vi "Main.vi"(11 "Module Admin":refnum<class "Delacor_lib_QMH_Module Admin.lvclass">) -> ()   [LabVIEW 2023, in "Panther Dashboard.lvlib"]
doc: "Panther Dashboard For DQMH®\n\nDeveloped and maintained by:\nPantherLAB\n\nMain Contributor- Developer:\n\n» Enrique Noé Arias\n\nBrainstorming & Code Reviews:\n\n» Matthias Baudot\n» Fabiola De La Cueva\n» Christopher Farmer\n» Cyril Gambini\n» Joerg Hampel\n» Olivier Jourdan\n» Cesar Muñoz\n» Darren Nattinger\n» Luis Orozco\n» Sam Taggart\n» Diego Torres\n\n<b>Note:</b> This VI was modified by the <b>Validate DQMH Module</b> tool to add a call to the Error Reported VI at the end of the 'Exit' MHL frame."
uses:
  Panther Dashboard.lvlib
  <vilib>/Delacor/Delacor QMH/Libraries/Module Admin_class/Delacor_lib_QMH_Module Admin.lvclass
  Module Data--cluster.ctl
  Maps List and refs--cluster.ctl
  <vilib>/National Instruments/Tree Map/Tree Map Data.ctl
  DQMH Modules Info--cluster.ctl
  Module type--enum.ctl
  Project References--cluster.ctl
  Selection Type--enum.ctl
  References Updated Argument--cluster.ctl
  Launch DQMH Scripting Tools Argument--cluster.ctl
  DQMH Tools Menu--enum.ctl
  <vilib>/Delacor/Delacor QMH/Libraries/Message Queue_class/Delacor_lib_QMH_Message Queue.lvclass/Delacor_lib_QMH_Message Queue.ctl
  Execute Default Event Request Argument--cluster.ctl
  Tree DQMH Selection Argument--cluster.ctl
  Expand Results Argument--cluster.ctl
  Scan DQMH Modules Argument--cluster.ctl
  Stop Argument--cluster.ctl
  Generate Project Documentation Argument--cluster.ctl
  Set App Theme Argument--cluster.ctl
  Show About Argument--cluster.ctl
  Update Module ID Argument--cluster.ctl
  Save Library Description Argument--cluster.ctl
  Save VI Description Argument--cluster.ctl
  Open Documentation Argument--cluster.ctl
  Save Project Documentation Argument--cluster.ctl
  Save Module Spec Argument--cluster.ctl
  Public VIs names--enum.ctl
  <vilib>/Delacor/Delacor QMH/Libraries/Module Admin_class/Delacor_lib_QMH_Module Admin.lvclass/Delacor_lib_QMH_Module Admin.ctl
  <vilib>/Delacor/Delacor QMH/Libraries/Message Queue_class/Delacor_lib_QMH_Enqueue Message (Single).vi
  <vilib>/Delacor/Delacor QMH/Libraries/Module Admin_class/Delacor_lib_QMH_Get External Launch.vi
  Panther Dashboard--global.vi
  <vilib>/Platform/browser.llb/Open URL in Default Browser (path).vi
  <vilib>/Utility/error.llb/Error Cluster From Error Code.vi
  <vilib>/ErrorRing/Error Ring.xnode
  <vilib>/Delacor/Delacor QMH/Libraries/Message Queue_class/Delacor_lib_QMH_Message Queue.lvclass
  <vilib>/National Instruments/Tree Map/Tree Map.lvlib
  <vilib>/Delacor/Delacor QMH/Libraries/Scripting API/DQMH_Scripting API.lvlib
  ContextHelp/ContextHelp.lvlib
panel:
  out "error out":errorcluster
  in  "Context Help Panther":bool caption="Doc Editor"
  in  "Add Event":bool
  in  "Remove Event":bool caption="Remove"
  in  "Convert Event":bool caption="Convert"
  in  "Rename Event":bool caption="Rename"
  in  "Add Helper Loop to Module":bool
  in  "Add New Module":bool caption="Add"
  in  "Rename Module":bool caption="Rename"
  in  "Validate Module":bool caption="Validate"
  in  "Create Module Template":bool caption="Template"
  in  "Add Unit Test Module":bool caption="Unit Test"
  in  "Create RT Tester Module":bool caption="RT Tester"
  in  "Open Antidoc Output":bool caption="Open"
  in  "Generate Antidoc":bool caption="Antidoc"
  in  "About Panther":bool caption="About"
  in  "Theme Panther":bool caption="Theme"
  in  "Projects":string(combo)
  in  "Targets":string(combo)
  in  "Save Module Spec":bool
  in  "Scan All":bool
  in  "Search":bool caption="Scan Project"
  in  "Include Dependencies":bool
  in  "Expand Results":bool
  in  "Module ID":i32=-1 min=-1 max=1000 step=1 format="Module ID %d"
  in  "Modules Tree":string(tree)
  out "antidoc":bool
  out "Panther Indicator":bool
  out "Process Indicator":bool
  out "Event Indicator":bool
  out "Status":string
  out "Progress":u16(slide) scale=-1.0..1.0
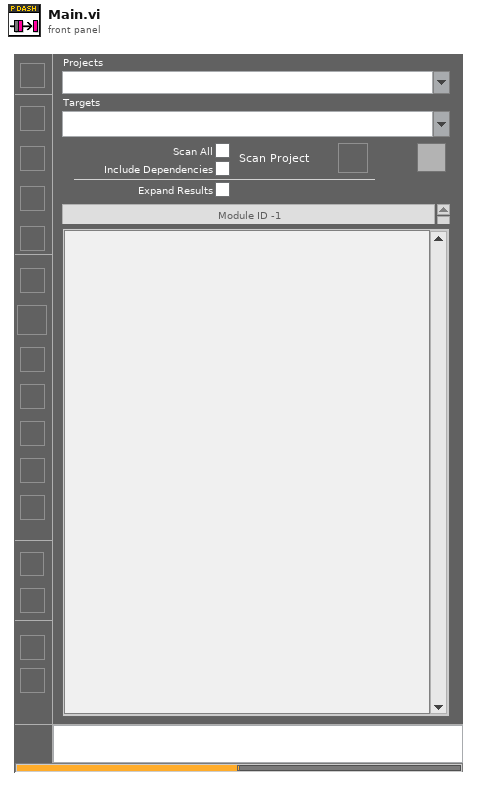
[diagram p1: front panel]
types:
  T1 = typedef "Panther Dashboard.lvlib/Broadcast Events--cluster.ctl" = cluster{"Module Did Init":refnum<user-event>, "Status Updated":refnum<user-event>, "Error Reported":refnum<user-event>, "Module Did Stop":refnum<user-event>, "Update Module Execution Status":refnum<user-event>, "References Updated":refnum<user-event>, "Projects Updated":refnum<user-event>, "Targets Updated":refnum<user-event>, "Progress updated":refnum<user-event>, "Scale Updated":refnum<user-event>, "Connector Pane Updated":refnum<user-event>, "Documentation Updated":refnum<user-event>, "Module Type Updated":refnum<user-event>, "Theme Updated":refnum<user-event>, "Project Description Updated":refnum<user-event>}
  T2 = typedef "Panther Dashboard.lvlib/Request Events--cluster.ctl" = cluster{"Stop Module":refnum<user-event>, "Show Panel":refnum<user-event>, "Hide Panel":refnum<user-event>, "Get Module Execution Status":refnum<user-event>, "Show Diagram":refnum<user-event>, "Scan DQMH Modules":refnum<user-event>, "Tree DQMH Selection":refnum<user-event>, "Open Module API Tester":refnum<user-event>, "Execute Default Event Request":refnum<user-event>, "Expand Results":refnum<user-event>, "Launch DQMH Scripting Tools":refnum<user-event>, "Generate Project Documentation":refnum<user-event>, "Set App Theme":refnum<user-event>, "Show About":refnum<user-event>, "Update Module ID":refnum<user-event>, "Save Library Description":refnum<user-event>, "Save VI Description":refnum<user-event>, "Open Documentation":refnum<user-event>, "Save Project Documentation":refnum<user-event>, "Register controls Mouse Enter":refnum<user-event>, "Save Module Spec":refnum<user-event>}
  T3 = typedef "ContextHelp.lvlib/Broadcast Events--cluster.ctl" = cluster{"Module Did Init":refnum<user-event>, "Status Updated":refnum<user-event>, "Error Reported":refnum<user-event>, "Module Did Stop":refnum<user-event>, "Update Module Execution Status":refnum<user-event>}
  T4 = typedef "Panther Dashboard.lvlib/Selection Type--enum.ctl" = enum16{"Module", "Public API", "Broadcast", "Request", "Request and Wait for Reply"}
  T5 = typedef "Panther Dashboard.lvlib/Module Data--cluster.ctl" = cluster{"Maps":T6, "DQMH Scan Results":T8, "Current Selection":cluster{"VI Ref":refnum<vi>, "DQMH Lib Ref":refnum<vi>}, "Module type":T9, "Module ID":i32, "Theme":bool, "Broadcast?":bool}
  T6 = typedef "Panther Dashboard.lvlib/Maps List and refs--cluster.ctl" = cluster{"Tree Map":T7, "References Map":map{string, refnum<vi>}}
  T7 = typedef "Tree Map.lvlib/Tree Map Data.ctl" = map{string, cluster{"Child Paths Set":set{string}, "Name":string, "Data":string, "Attributes":map{string, string}}}
  T8 = typedef "Panther Dashboard.lvlib/DQMH Modules Info--cluster.ctl" = cluster{"All DQMH Modules Refs":refnum<vi>[], "All Modules Descriptions":string[], "All Modules type":T9[], "Project References":T10, "Dependencies":bool[]}
  T9 = typedef "Panther Dashboard.lvlib/Module type--enum.ctl" = enum16{"Singleton", "Cloneable"}
  T10 = typedef "Panther Dashboard.lvlib/Project References--cluster.ctl" = cluster{"Project Ref":refnum<vi>, "Project Name":string, "Target":refnum<vi>, "App Ref":refnum<vi>}
  T11 = typedef "Panther Dashboard.lvlib/References Updated Argument--cluster.ctl" = cluster{"Modules":refnum<vi>[], "Modules Types":T9[], "Application Instance":refnum<vi>, "Dependencies":bool[]}
  T12 = enum8{"Enabled", "Disabled", "Disabled and Grayed Out"}
  T13 = typedef "Panther Dashboard.lvlib/Launch DQMH Scripting Tools Argument--cluster.ctl" = cluster{"Scripting Tool":T14}
  T14 = typedef "Panther Dashboard.lvlib/DQMH Tools Menu--enum.ctl" = enum16{"Create New DQMH Event", "Remove DQMH Event", "Convert DQMH Event", "Rename DQMH Event", "Add New DQMH Module", "Create RT Tester", "Rename DQMH Module", "Validate DQMH Module", "Create DQMH Module Template", "New DQMH  Unit Test", "Add Helper Loop to DQMH Module"}
  T15 = typedef "Panther Dashboard.lvlib/Execute Default Event Request Argument--cluster.ctl" = cluster{"Event Name":string}
  T16 = typedef "Panther Dashboard.lvlib/Tree DQMH Selection Argument--cluster.ctl" = cluster{"Tree DQMH Sel":string}
  T17 = typedef "Panther Dashboard.lvlib/Expand Results Argument--cluster.ctl" = cluster{"Expand?":bool}
  T18 = typedef "Panther Dashboard.lvlib/Scan DQMH Modules Argument--cluster.ctl" = cluster{"Include Dependencies":bool, "Scan All":bool, "Project":string, "Target":string}
  T19 = enum32{"invalid lock state", "Not Locked", "Locked (No Password)", "Password-protected"}
  T20 = typedef "Panther Dashboard.lvlib/Stop Argument--cluster.ctl" = cluster{"Origin":string, "Exit via Stop Module Req?":bool, "Wait for Module to stop?":bool}
  T21 = typedef "Panther Dashboard.lvlib/Generate Project Documentation Argument--cluster.ctl" = cluster{"Boolean":bool}
  T22 = typedef "Panther Dashboard.lvlib/Set App Theme Argument--cluster.ctl" = cluster{"Theme":bool}
  T23 = typedef "Panther Dashboard.lvlib/Show About Argument--cluster.ctl" = cluster{"Boolean":bool}
  T24 = typedef "Panther Dashboard.lvlib/Update Module ID Argument--cluster.ctl" = cluster{"New ID":i32}
  T25 = typedef "Panther Dashboard.lvlib/Save Library Description Argument--cluster.ctl" = cluster{"Library Description":string}
  T26 = typedef "Panther Dashboard.lvlib/Save VI Description Argument--cluster.ctl" = cluster{"VI Description":string}
  T27 = typedef "Panther Dashboard.lvlib/Open Documentation Argument--cluster.ctl" = cluster{"Boolean":bool}
  T28 = typedef "Panther Dashboard.lvlib/Save Project Documentation Argument--cluster.ctl" = cluster{"Project Description":string}
  T29 = typedef "Panther Dashboard.lvlib/Save Module Spec Argument--cluster.ctl" = cluster{"Boolean":bool}
  T30 = typedef "Panther Dashboard.lvlib/Public VIs names--enum.ctl" = enum16{"Start Module.vi", "Synchronize Module Events.vi", "Obtain Broadcast Events for Registration.vi", "Null Broadcast Events--constant.vi", "Stop Module.vi"}
  T31 = enum32{"Invalid", "Standard", "Closed", "Hidden", "Minimized", "Maximized"}
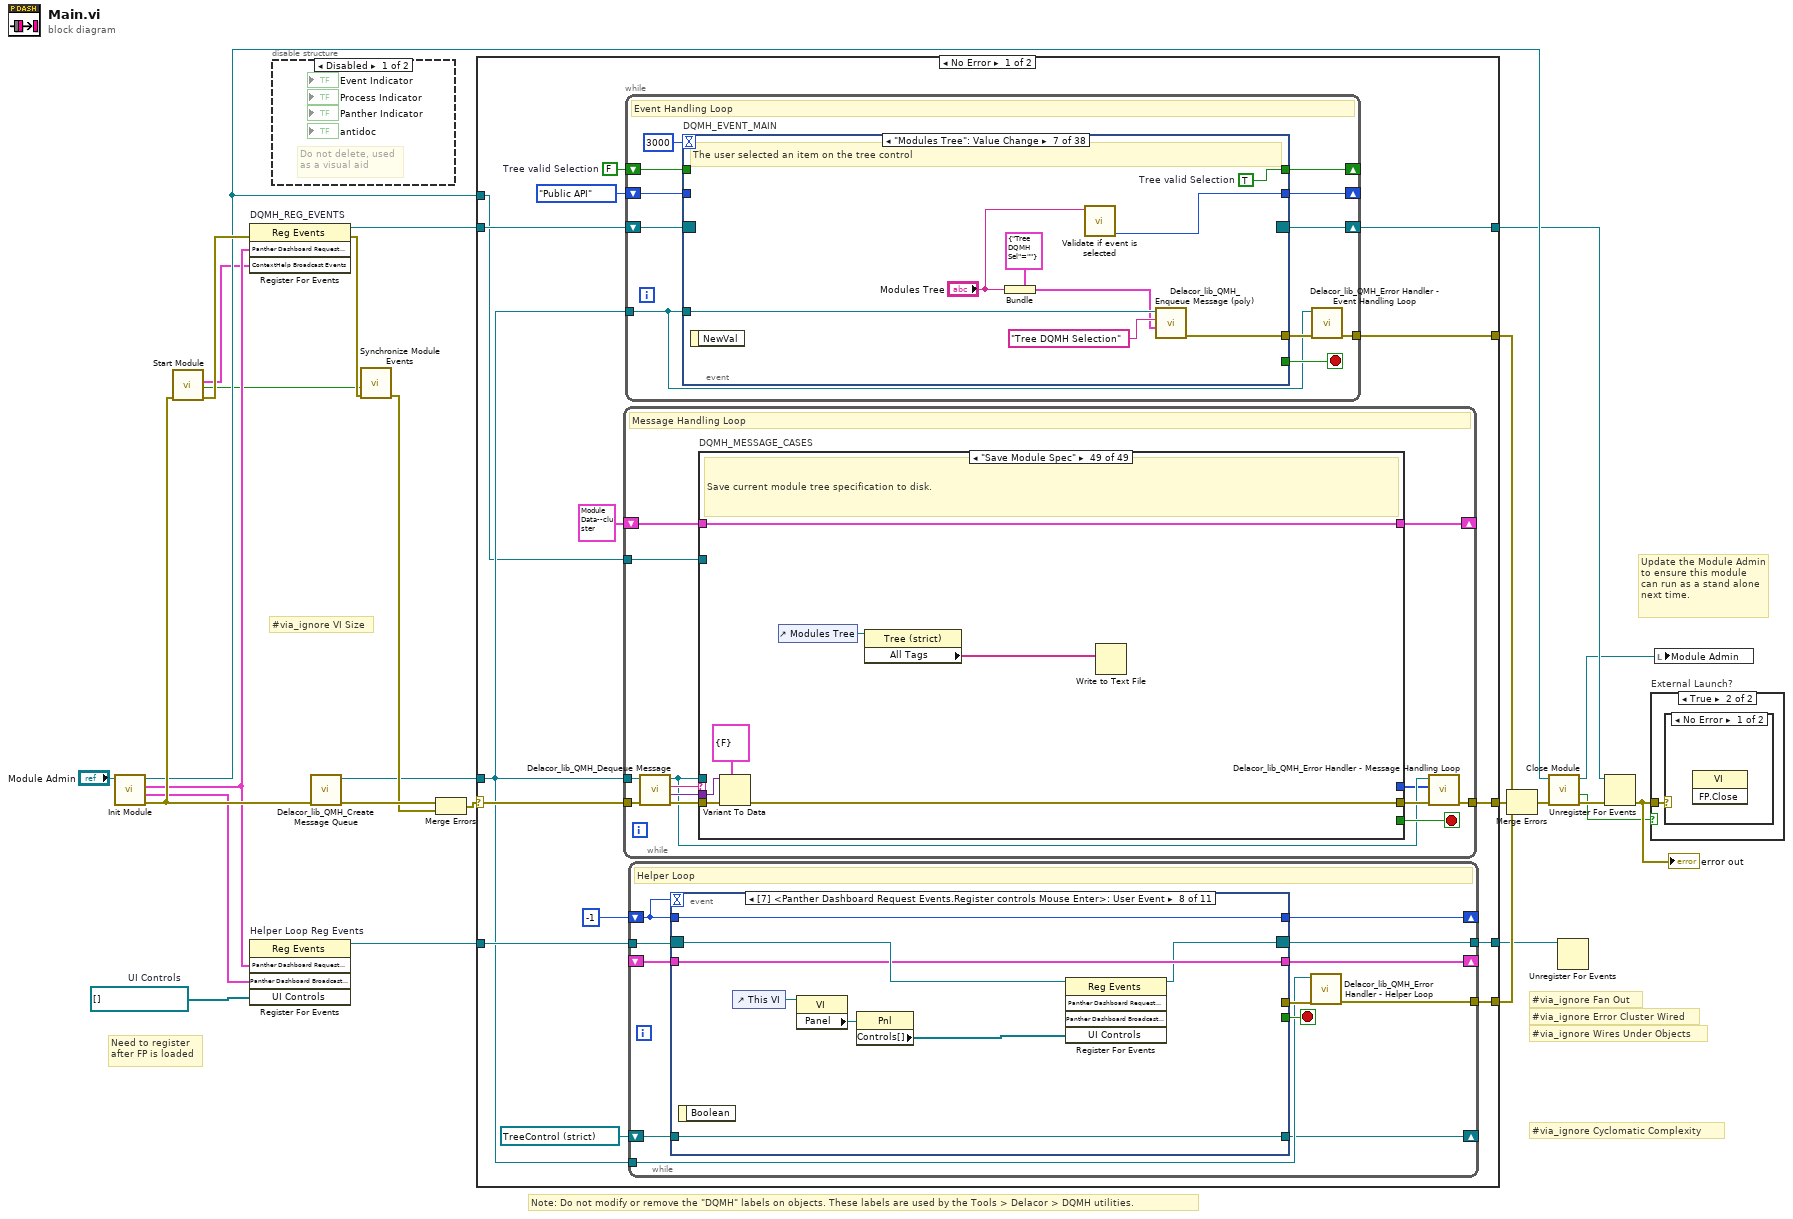
[diagram p0: block diagram]
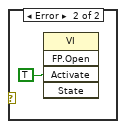
[diagram p4: hidden frame]
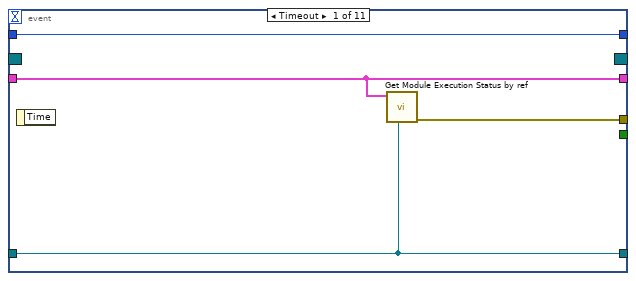
[diagram p5: hidden frame]
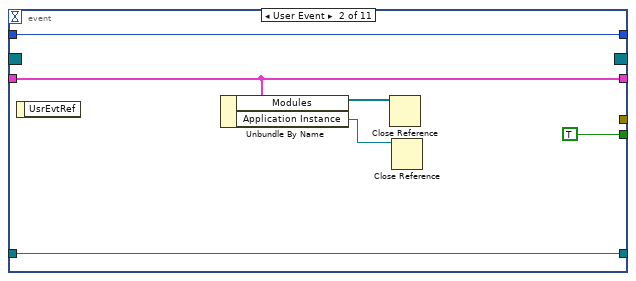
[diagram p6: hidden frame]
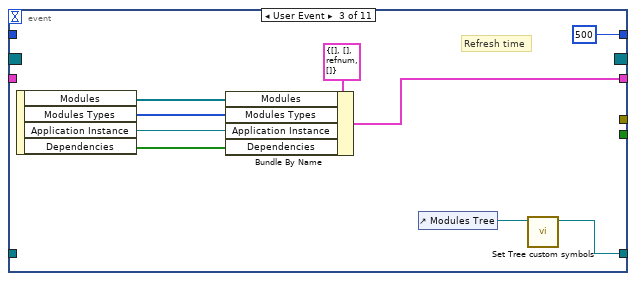
[diagram p7: hidden frame]
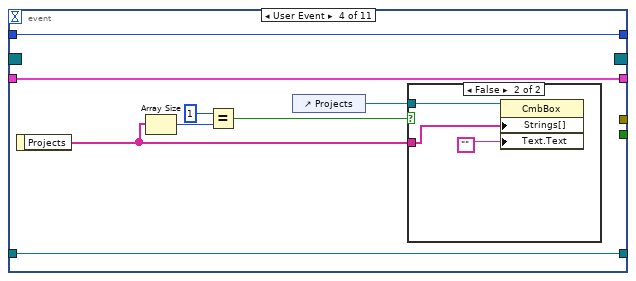
[diagram p8: hidden frame]
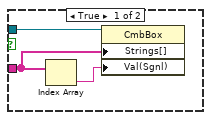
[diagram p9: hidden frame]
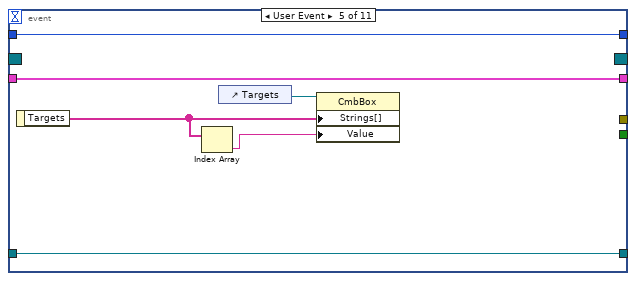
[diagram p10: hidden frame]
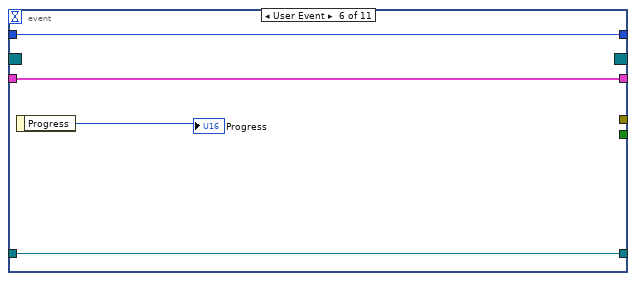
[diagram p11: hidden frame]
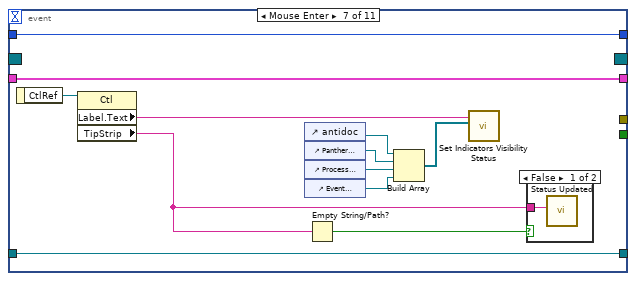
[diagram p12: hidden frame]
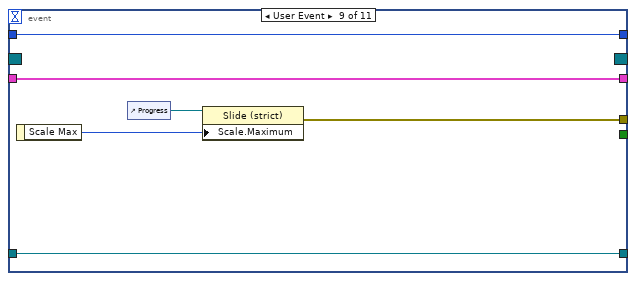
[diagram p14: hidden frame]
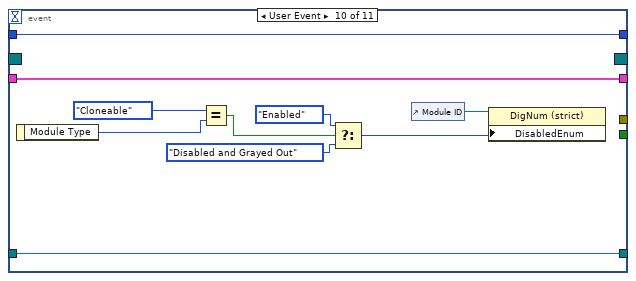
[diagram p15: hidden frame]
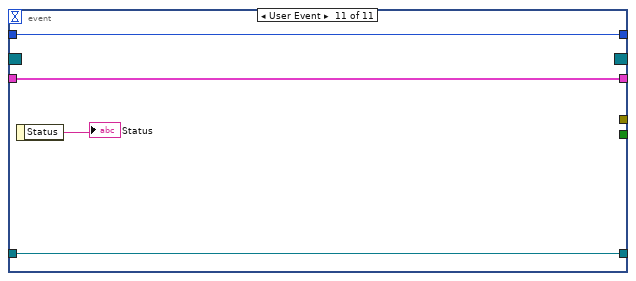
[diagram p16: hidden frame]
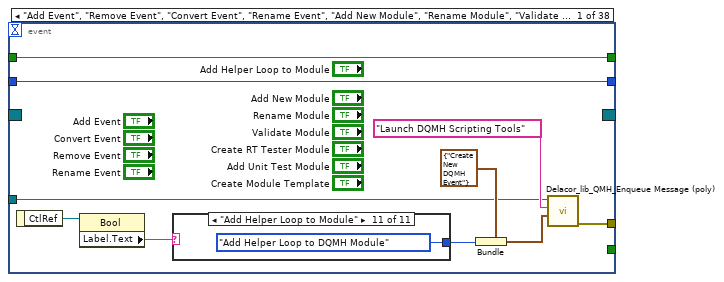
[diagram p17: hidden frame]
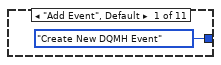
[diagram p18: hidden frame]
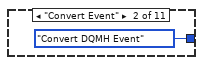
[diagram p19: hidden frame]
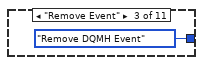
[diagram p20: hidden frame]
diagram:
  w1 = refnum<vi>[] []  # UI Controls
  # "Need to register\nafter FP is loaded"
  # "#via_ignore VI Size"
  # "#via_ignore Fan Out"
  # "#via_ignore Cyclomatic Complexity"
  # "#via_ignore Wires Under Objects"
  # "#via_ignore Error Cluster Wired"
  # "Note: Do not modify or remove the \"DQMH\" labels on objects. These labels are used by the Tools > Delacor > DQMH utilities."
  # "Update the Module Admin to ensure this module can run as a stand alone next time."
  n1 = call "Init Module.vi"("Singleton Module Admin in"="Module Admin") -> ("error out"=w15:errorcluster, "Panther Dashboard Broadcast Events"=w4:T1, "Panther Dashboard Request Events"=w5:T2, "Singleton Module Admin out"=w14:refnum<class "Delacor_lib_QMH_Module Admin.lvclass">)  [unwired: 7 in]
  n2 = call "Start Module.vi"("error in"=w15) -> ("error out"=w17:errorcluster, "Wait for Event Sync?"=w3:bool, "ContextHelp Broadcast Events"=w2:T3)  [unwired: 7 in, 1 out]
  n3 = register-events "DQMH_REG_EVENTS"(error in=w17, w5, w2) -> (reference out=w12:refnum<event-registration>, error out=w18:errorcluster)  [unwired: 1 in]
  n4 = register-events "Helper Loop Reg Events"(w5, w4, w1) -> (reference out=w7:refnum<event-registration>)  [unwired: 2 in, 1 out]
  n5 = disable-structure shown="Disabled" {
    frame Disabled {
      # "Do not delete, used\nas a visual aid"
    }
    frame Enabled {
    }
  }
  n6 = call <vilib>:"Delacor_lib_QMH_Create Message Queue.vi"("error in"=w15) -> ("error out"=w21:errorcluster, "Message Queue"=w11:refnum<class "Delacor_lib_QMH_Message Queue.lvclass">)  [unwired: 9 in]
  n7 = call "Synchronize Module Events.vi"("error in"=w18, "Wait for Event Sync?"=w3) -> ("error out"=w16:errorcluster)  [unwired: 9 in]
  n8 = Merge Errors(w21, w16) -> (w20:errorcluster)
  n9 = case shown="No Error" w20 {
    selector: w20 -> [w39 w924]
    tunnel: [w41 w923] -> w26
    tunnel: [w37 w922] -> w13
    tunnel: w12 -> [w35 w922]
    tunnel: w11 -> [w31 w918]
    tunnel: [w40 _] -> w24
    tunnel: w14 -> [w28 w919]
    tunnel: w7 -> [w34 w917]
    tunnel: [w33 w917] -> w6
    tunnel: [w38 _] -> w19
    frame No Error {
      w30 = FALSE  # Tree valid Selection
      n10 = while {
        tunnel: w31 -> [w466]
        shift-right: [w470] -> _
        shift-left: T5 {"Maps"={"Tree Map"={}, "References Map"={}}, "DQMH Scan Results"={"All DQMH Modules Refs"=[], "All Modules Descriptions"=[], "All Modules type"=[], "Project References"={"Project Ref"=refnum, "Project Name"="", "Target"=refnum, "App Ref"=refnum}, "Dependencies"=[]}, "Current Selection"={"VI Ref"=refnum, "DQMH Lib Ref"=refnum}, "Module type"=enum."Singleton", "Module ID"=0, "Theme"=FALSE, "Broadcast?"=FALSE} ("Data Cluster") -> [w471]
        tunnel: w39 -> [w474]
        tunnel: [w472] -> w41
        tunnel: w28 -> [w464]
        stop <- w469 stop-if-true
        # "Message Handling Loop"
        n11 = call-dynamic "Delacor_lib_QMH_Dequeue Message.vi"("error in"=w474, "Message Queue in"=w466) -> ("error out"=w473:errorcluster, "Message Data"=w467:variant, "Message"=w468:string, "Message Queue out"=w465:refnum<class "Delacor_lib_QMH_Message Queue.lvclass">)  [unwired: 6 in]
        n12 = case "DQMH_MESSAGE_CASES" shown="\"Save Module Spec\"" w468 {
          selector: w468 -> [_ _ _ _ w525 _ _ _ _ _ _ _ _ _ _ _ _ _ _ _ _ _ _ _ _ _ _ _ _ _ _ _ _ _ _ _ _ _ _ _ _ _ _ _ _ _ _ w896 _]
          tunnel: w465 -> [_ _ _ _ _ _ _ _ _ _ _ _ _ _ _ _ _ _ _ _ _ _ _ _ _ _ _ _ _ _ _ _ _ _ _ _ _ _ _ _ _ _ _ _ _ w865 w888 _ _]
          tunnel: w473 -> [w496 w501 w510 w522 w530 w537 w544 w551 w560 w567 w573 w579 w586 w593 w598 w604 w606 w613 w615 w620 w634 w647 w669 w676 w682 w687 w693 w700 w707 w720 w722 w732 w741 w749 w764 w766 w771 w781 w798 w807 w817 w831 w849 w860 w862 w872 w894 w898 w915]
          tunnel: [w490 w501 w508 w521 w528 w536 w544 w551 w559 w566 w572 w578 w585 w592 w599 w603 w606 w613 w615 w621 w632 w646 w670 w677 w681 w686 w692 w699 w706 w718 w722 w730 w737 w748 w763 w766 w770 w780 w798 w805 w815 w829 w848 w858 w862 w868 w891 w899 w914] -> w475
          tunnel: w471 -> [w476 w500 w505 w520 w527 w534 w543 w550 w558 w565 w571 w577 w584 w591 w597 w602 w605 w612 w614 w619 w627 w644 w668 w674 w680 w685 w691 w698 w705 w709 w721 w729 w736 w747 w759 w765 w769 w778 w797 w801 w810 w823 w838 w854 w861 w867 w880 w897 w911]
          tunnel: [w487 w500 w504 w519 w527 w534 w543 w550 w558 w565 w571 w577 w584 w591 w597 w602 w605 w612 w614 w619 w627 w644 w668 w674 w680 w685 w691 w696 w705 w709 w721 w724 w736 w743 w755 w765 w769 w778 w797 w801 w808 w822 w838 w854 w861 w867 w880 w897 w911] -> w470
          tunnel: [_ _ _ _ _ _ _ _ _ _ _ _ _ _ _ _ _ _ _ _ _ _ _ _ _ _ _ _ _ _ _ _ _ _ _ _ _ _ _ _ _ _ _ _ _ _ w887 _ _] -> w469
          tunnel: w467 -> [_ _ w507 _ w526 _ _ _ _ _ _ _ _ _ _ _ _ _ _ _ w630 _ _ _ _ _ _ w697 w704 w717 _ w728 w735 w746 w762 _ _ _ _ w803 w813 w827 w847 w857 _ w866 w886 _ w913]
          tunnel: w464 -> [w488 _ _ _ _ _ _ _ _ _ _ _ _ _ _ _ _ _ _ _ _ _ _ _ _ _ _ _ _ _ _ _ _ _ _ _ _ _ _ _ _ _ _ _ _ w864 w881 _ _]
          tunnel: [_ _ _ _ _ _ _ _ _ _ _ _ _ _ _ _ _ _ _ _ _ i32[] [5000, 1026, 43] ("specific error code to clear (0: all)") _ _ _ _ _ _ _ _ _ _ _ _ _ _ _ _ _ _ _ _ _ _ _ _ _ _ _] -> w463
          frame "Initialize" {
            w478 = "Panther Dashboard for DQMH" ("format string")
            # "Initialize - Any operation that needs to be done before the module can receive messages. Synchronize Caller Events.vi will inform Start Module.vi that the module has launched and is ready to receive messages. Module Did Init.vi will broadcast that the module initialized."
            n13 = call "Synchronize Caller Events.vi"("error in (no error)"=w496, "Singleton Module Admin in"=w488) -> ("error out"=w495:errorcluster)  [unwired: 8 in, 1 out]
            n14 = property on="Modules Tree" class="Tree (strict)"("Allow Item Drag"=TRUE ("Drag/Drop:Allow Dragging"), "SelColor"=u32 8355711) -> ()  [unwired: 2 in, 2 out]
            n15 = call "Module Name--constant.vi"() -> ("Module Name"=w485:string)  [unwired: 11 in]
            n16 = call "Module Did Init.vi"("error in (no error)"=w495, "Initialized?"=TRUE, "Origin"=w485) -> ("error out"=w494:errorcluster)  [unwired: 8 in]
            n17 = control-ref of="Projects"() -> (w481:refnum<vi>)
            n18 = call "Scan For App Projects.vi"("error in"=w494, "Init?"=TRUE, "Projects Ref"=w481) -> ("error out"=w493:errorcluster)  [unwired: 8 in]
            n19 = call "Read Theme from Config.vi"("error in"=w493) -> ("error out"=w492:errorcluster, "Theme"=w477:bool)  [unwired: 9 in]
            n20 = local write "Theme Panther"(w477) -> ()
            n21 = call "Set App Theme.vi"("error in"=w492, "Theme"=w477) -> ("error out"=w491:errorcluster)  [unwired: 9 in]
            n22 = control-ref of="This VI"() -> (w479:refnum<vi>)
            n23 = disable-structure shown="Disabled" {
              disable-tunnel: [w499 _] -> w489
              disable-tunnel: w479 -> [w498 _]
              disable-tunnel: w478 -> [w497 _]
              frame Disabled {
                n24 = call "Set Panel Initial State.vi"("Title"=w497, "Main Vi Ref"=w498) -> ("error out"=w499:errorcluster)  [unwired: 9 in]
              }
              frame Enabled {
              }
            }
            n25 = Bundle By Name(cluster=w476, "Module ID"=-1) -> (w487:T5)
            n26 = call "Status Updated.vi"("Status"=w478) -> ()  [unwired: 10 in, 1 out]
            n27 = Merge Errors(w489, w491) -> (w490:errorcluster)
          }
          frame "--------MODULE-----------" {
          }
          frame "Scan DQMH Modules" {
            # "Scan DQMH Modules in the project and fill 2 maps one with the Vi References and the another one with the list of DQMH modules on the project"
            n28 = Variant To Data(error in=w510, type=T18 {"Include Dependencies"=FALSE, "Scan All"=FALSE, "Project"="", "Target"=""} ("Scan DQMH Modules Argument"), Variant=w507) -> (data=w502:T18, error out=w509:errorcluster)
            n29 = call <vilib>:"Set Busy.vi"("error in (no error)"=w509) -> ()  [unwired: 9 in, 2 out]
            n30 = control-ref of="Modules Tree"() -> (w503:refnum<vi>)
            n31 = call "Scan DQMH Modules and create Maps.vi"("TreeControl in"=w503, "Data Cluster In"=w505, "error in"=w509, "Scan DQMH Modules Argument"=w502) -> ("error out"=w508:errorcluster, "Data Cluster Out"=w504:T5)  [unwired: 6 in]
            n32 = call <vilib>:"Unset Busy.vi"("error in (no error)"=w508) -> ()  [unwired: 10 in, 1 out]
          }
          frame "Refresh Module" {
            # "User right click a module and selected Refresh module"
            n33 = Unbundle By Name(w520) -> ("DQMH Scan Results.Project References.App Ref"=w513:refnum<vi>, "Current Selection.DQMH Lib Ref"=w514:refnum<vi>, "Maps.Tree Map"=w516:T7, "Maps.References Map"=w515:map{string, refnum<vi>})
            n34 = local read "Expand Results"() -> (w512:bool)
            n35 = control-ref of="Modules Tree"() -> (w511:refnum<vi>)
            n36 = call "Refresh Current DQMH Module.vi"("TreeControl in"=w511, "App Ref"=w513, "Expand Results"=w512, "DQMH Lib Ref"=w514, "error in"=w522, "References Map"=w515, "Tree Map In"=w516) -> ("error out"=w521:errorcluster, "map ref out"=w518:map{string, refnum<vi>}, "Tree Map out"=w517:T7)  [unwired: 2 in]
            n37 = Bundle By Name(cluster=w520, "Maps.Tree Map"=w517, "Maps.References Map"=w518) -> (w519:T5)
          }
          frame "Refresh Targets" {
            # "When the User selects a Project triggers this task to scan all the targets available"
            n38 = Variant To Data(error in=w530, type=w525, Variant=w526) -> (data=w524:string, error out=w529:errorcluster)
            n39 = call "Get all Targets.vi"("error in"=w529, "Project Selection"=w524) -> ("error out"=w528:errorcluster, "Targets"=w523:string[])  [unwired: 8 in]
            n40 = call "Targets Updated.vi"("Targets"=w523) -> ()  [unwired: 10 in, 1 out]
          }
          frame "Drag VI" {
            # "This is the functionality alowing drag and drop the current selection to your code, you can edit DQMH code using panther Dashboard as it was the Project Explorer"
            n41 = Unbundle By Name(w534) -> ("DQMH Scan Results.Project References.App Ref"=w533:refnum<vi>, "DQMH Scan Results.Project References.Target"=w532:refnum<vi>, "Current Selection.VI Ref"=w531:refnum<vi>)
            n42 = call "Drop Event into subVI.vi"("Current Selection.VI Ref"=w531, "Target"=w532, "App Ref"=w533) -> ("error out"=w535:errorcluster)  [unwired: 8 in]
            n43 = Merge Errors(w535, w537) -> (w536:errorcluster)
          }
          frame "Where is this module being Launched?" {
            # "Find all the VIS calling the Start Module.vi of the selected module library"
            n44 = Unbundle By Name(w543) -> ("Theme"=w542:bool, "DQMH Scan Results.Project References.App Ref"=w541:refnum<vi>, "DQMH Scan Results.Project References.Target"=w540:refnum<vi>, "Current Selection.DQMH Lib Ref"=w539:refnum<vi>)
            n45 = call "Find some Public API VI.vi"("Theme"=w542, "Framework VI to Find"=Public_VIs_names--enum."Start Module.vi", "Library in"=w539, "Target"=w540, "App Ref"=w541) -> ()  [unwired: 7 in]
          }
          frame "Where is this module being Stopped?" {
            # "Find all the VIS calling the Obtain broadcast events for registration of the selected module library"
            n46 = Unbundle By Name(w550) -> ("Theme"=w548:bool, "DQMH Scan Results.Project References.App Ref"=w547:refnum<vi>, "DQMH Scan Results.Project References.Target"=w546:refnum<vi>, "Current Selection.DQMH Lib Ref"=w545:refnum<vi>)
            n47 = call "Find some Public API VI.vi"("Theme"=w548, "Framework VI to Find"=Public_VIs_names--enum."Stop Module.vi", "Library in"=w545, "Target"=w546, "App Ref"=w547) -> ()  [unwired: 7 in]
          }
          frame "Open Module API Tester" {
            # "If nothing selected use the first DQMH module"
            # "Open the API Tester from the current DQMH Module Selected"
            n48 = Unbundle By Name(w558) -> ("DQMH Scan Results.Project References.App Ref"=w557:refnum<vi>, "DQMH Scan Results.All DQMH Modules Refs"=w556:refnum<vi>[], "Current Selection.DQMH Lib Ref"=w552:refnum<vi>)
            n49 = Index Array(array=w556) -> (element=w554:refnum<vi>)  [unwired: 1 in]
            n50 = Not A Number/Path/Refnum?(number/path/refnum=w552) -> (NaN/Path/Refnum?=w555:bool)
            n51 = Select(t=w554, s=w555, f=w552) -> (s? t:f=w553:refnum<vi>)
            n52 = call "Open API Tester.vi"("error in"=w560, "DQMH Library Ref"=w553, "Application Instance"=w557) -> ("error out"=w559:errorcluster)  [unwired: 8 in]
          }
          frame "Create Custom --error.vi" {
            n53 = Unbundle By Name(w565) -> ("Module type"=w561:T9, "Current Selection.DQMH Lib Ref"=w564:refnum<vi>, "Theme"=w563:bool, "DQMH Scan Results.Project References.App Ref"=w562:refnum<vi>)
            n54 = call "Error Code Dialog.vi"("Module type"=w561, "error in"=w567, "App Ref"=w562, "Theme"=w563, "Library in"=w564) -> ("error out"=w566:errorcluster)  [unwired: 6 in]
          }
          frame "Create Custom --constant.vi" {
            n55 = Unbundle By Name(w571) -> ("Current Selection.DQMH Lib Ref"=w570:refnum<vi>, "Theme"=w569:bool, "DQMH Scan Results.Project References.App Ref"=w568:refnum<vi>)
            n56 = call "Custom Constant Dialog.vi"("error in"=w573, "App Ref"=w568, "Theme"=w569, "Library in"=w570) -> ("error out"=w572:errorcluster)  [unwired: 7 in]
          }
          frame "Edit 'Module Name--constant.vi' value" {
            # "Sometimes we need to update or modify the 'Module Name--constant.vi' value and we need to go to this vi, open it's block diagram and change the constant value, close the vi and save it, this script does exactly that."
            n57 = Unbundle By Name(w577) -> ("Theme"=w574:bool, "DQMH Scan Results.Project References.App Ref"=w576:refnum<vi>, "Current Selection.DQMH Lib Ref"=w575:refnum<vi>)
            n58 = call "Script Edit Module Name.vi"("Theme"=w574, "error in"=w579, "Library in"=w575, "App Ref"=w576) -> ("error out"=w578:errorcluster)  [unwired: 7 in]
          }
          frame "Edit 'Module Timeout--constant.vi' value" {
            w580 = FALSE  # Restore to Default
            # "Sometimes we need to update or modify the 'Module Name--constant.vi' value and we need to go to this vi, open it's block diagram and change the constant value, close the vi and save it, this script does exactly that."
            n59 = Unbundle By Name(w584) -> ("Theme"=w581:bool, "DQMH Scan Results.Project References.App Ref"=w583:refnum<vi>, "Current Selection.DQMH Lib Ref"=w582:refnum<vi>)
            n60 = call "Script Module Timeout.vi"("Restore to Default"=w580, "Theme"=w581, "error in"=w586, "Library in"=w582, "App Ref"=w583) -> ("error out"=w585:errorcluster)  [unwired: 6 in]
          }
          frame "Restore Timeout to Default (5000ms)" {
            w587 = TRUE  # Restore to Default
            # "Restore Timeout to Default DQMH Framework value (5000ms)"
            n61 = Unbundle By Name(w591) -> ("Theme"=w588:bool, "DQMH Scan Results.Project References.App Ref"=w590:refnum<vi>, "Current Selection.DQMH Lib Ref"=w589:refnum<vi>)
            n62 = call "Script Module Timeout.vi"("Restore to Default"=w587, "Theme"=w588, "error in"=w593, "Library in"=w589, "App Ref"=w590) -> ("error out"=w592:errorcluster)  [unwired: 6 in]
          }
          frame "Find Module in project" {
            # "Find the selected module in project explorer"
            n63 = Unbundle By Name(w597) -> ("Current Selection.DQMH Lib Ref"=w596:refnum<vi>, "DQMH Scan Results.Project References.Project Ref"=w595:refnum<vi>, "DQMH Scan Results.All DQMH Modules Refs"=w594:refnum<vi>[])
            n64 = call "Find Library in Project.vi"("error in"=w598, "DQMH Modules Refs"=w594, "Project Ref"=w595, "DQMH Lib Ref"=w596) -> ("error out"=w599:errorcluster)  [unwired: 7 in]
          }
          frame "Open File Library on Disk" {
            # "Open current Module Library selection on the file system"
            n65 = Unbundle By Name(w602) -> ("Current Selection.DQMH Lib Ref"=w601:refnum<vi>)
            n66 = property class="Library"(reference=w601) -> ("Path"=w600:path)  [unwired: 1 in, 2 out]
            n67 = call "Open File on Disk.vi"("error in"=w604, "file or directory path"=w600) -> ("error out"=w603:errorcluster)  [unwired: 9 in]
          }
          frame "---------BROADCASTS---------" {
          }
          frame "Find Code registered to this module's broadcasts" {
            # "Find all the VIS calling the Obtain broadcast events for registration of the selected module library"
            n68 = Unbundle By Name(w612) -> ("Theme"=w610:bool, "DQMH Scan Results.Project References.App Ref"=w609:refnum<vi>, "DQMH Scan Results.Project References.Target"=w608:refnum<vi>, "Current Selection.DQMH Lib Ref"=w607:refnum<vi>)
            n69 = call "Find some Public API VI.vi"("Theme"=w610, "Framework VI to Find"=Public_VIs_names--enum."Obtain Broadcast Events for Registration.vi", "Library in"=w607, "Target"=w608, "App Ref"=w609) -> ()  [unwired: 7 in]
          }
          frame "---------REQUEST--------------" {
          }
          frame "Locate Event on Main" {
            # "Find the selected event vi on the owing DQMH Module, if it is a reques we highlight its frame, if it is a broadcast we highlight where the broadcast is being triggered"
            n70 = Unbundle By Name(w619) -> ("DQMH Scan Results.Project References.App Ref"=w617:refnum<vi>, "Current Selection.VI Ref"=w618:refnum<vi>, "Broadcast?"=w616:bool)
            n71 = call "Find Event Frame.vi"("error in"=w620, "Broadcast?"=w616, "VI in"=w618, "Application Instance"=w617) -> ("error out"=w621:errorcluster)  [unwired: 7 in]
          }
          frame "Execute Default Event Request" {
            # "Execute Default Event"
            n72 = Variant To Data(error in=w634, type=T15 {"Event Name"=""} ("Execute Default Event Request Argument"), Variant=w630) -> (data=w628:T15, error out=w633:errorcluster)
            n73 = Unbundle By Name(w627) -> ("DQMH Scan Results.Project References.App Ref"=w626:refnum<vi>, "Current Selection.DQMH Lib Ref"=w625:refnum<vi>, "Module ID"=w623:i32, "Module type"=w622:T9)
            n74 = Unbundle By Name(w628) -> ("Event Name"=w624:string)
            n75 = call "Execute Default event.vi"("Module type"=w622, "Module ID"=w623, "Event"=w624, "DQMH Library Ref"=w625, "application Instance"=w626) -> ("error out"=w631:errorcluster)  [unwired: 6 in]
            n76 = Merge Errors(w633, w631) -> (w632:errorcluster)
          }
          frame "Search for Event Callers / listeners" {
            # "1026-Invalid Ref\n43- Operation\n canceled by user\n5000- something\nrandom happening\non DQMH Scripting\nAPI"
            # "Search for this event callers"
            n77 = Unbundle By Name(w644) -> ("DQMH Scan Results.Project References.Project Ref"=w638:refnum<vi>, "Current Selection.VI Ref"=w643:refnum<vi>, "Theme"=w635:bool, "Broadcast?"=w636:bool)
            n78 = Select(t="Searching code registered to broadcast selection" ("Status"), s=w636, f="Searching for Event Callers" ("Status")) -> (s? t:f=w639:string)
            n79 = call "Status Updated.vi"("error in (no error)"=w647, "Status"=w639) -> ("error out"=w645:errorcluster)  [unwired: 9 in]
            n80 = case shown="True" w636 {
              tunnel: w645 -> [w652 w659]
              tunnel: [w651 w658] -> w646
              tunnel: w643 -> [w650 w655]
              tunnel: [w649 w657] -> w642
              tunnel: w638 -> [w648 w656]
              frame False {
                # "Requests"
                n81 = call <vilib>:"Get Callers of Request VI in Project.vi"("error in"=w652, "Request VI"=w650, "Project"=w648) -> ("error out"=w651:errorcluster, "Request VI Callers"=w649:refnum<vi>[])  [unwired: 7 in]
              }
              frame True {
                # "Broadcast"
                n82 = Two Button Dialog(message="This is an exhaustive task that can take up to minutes, do you wish to continue?") -> (T button?=w654:bool)  [unwired: 2 in]
                n83 = case shown="True" w654 {
                  tunnel: w659 -> [w660 w665]
                  tunnel: [w660 w664] -> w658
                  tunnel: [_ w663] -> w657
                  tunnel: w656 -> [_ w662]
                  tunnel: w655 -> [_ w661]
                  frame False {
                  }
                  frame True {
                    n84 = call <vilib>:"Get VIs Registered for Broadcast in Project.vi"("error in"=w665, "Broadcast VI"=w661, "Project"=w662) -> ("error out"=w664:errorcluster, "VIs Registered for Broadcast"=w663:refnum<vi>[])  [unwired: 7 in]
                  }
                }
              }
            }
            n85 = call <vilib>:"Set Busy.vi"("error in (no error)"=w645) -> ()  [unwired: 9 in, 2 out]
            n86 = call <vilib>:"Unset Busy.vi"("error in (no error)"=w646) -> ()  [unwired: 10 in, 1 out]
            n87 = call "Start Call to results window.vi"("Find Broadcast?"=w636, "Request VI Callers"=w642, "Event"=w643, "Theme"=w635) -> ()  [unwired: 8 in]
          }
          frame "Open VI on Disk" {
            # "Open current event selection on the file system"
            n88 = Unbundle By Name(w668) -> ("Current Selection.VI Ref"=w667:refnum<vi>)
            n89 = property class="VI"(reference=w667) -> ("Path"=w666:path)  [unwired: 1 in, 2 out]
            n90 = call "Open File on Disk.vi"("error in"=w669, "file or directory path"=w666) -> ("error out"=w670:errorcluster)  [unwired: 9 in]
          }
          frame "Open Event Arguments" {
            # "Open The event selected DQMH Arguments, also open the Event BD to do edits on it"
            n91 = Unbundle By Name(w674) -> ("Current Selection.VI Ref"=w673:refnum<vi>)
            n92 = property on="Property Node" class="VI"(reference=w673, error in=w676, "BDWin.Open"=TRUE ("Block Diagram Window:Open")) -> (reference out=w671:refnum<vi>, error out=w675:errorcluster)
            n93 = call "Open Event Arguments.vi"("error in"=w675, "VI Refnum"=w671) -> ("error out"=w677:errorcluster)  [unwired: 9 in]
          }
          frame "Set Custom Timeout" {
            n94 = Unbundle By Name(w680) -> ("Theme"=w678:bool, "Current Selection.VI Ref"=w679:refnum<vi>)
            n95 = call "Script Request and Wait For Reply Custom Timeout.vi"("error in"=w682, "VI Ref"=w679, "Theme"=w678) -> ("error out"=w681:errorcluster)  [unwired: 8 in]
          }
          frame "Restore to Module's Timeout" {
            # "The requests and wait for reply utilize a notifier created on the fly to get the module's answer (Reply), there is a Wait for Notifier funtion with a timeout input, by default all the DQMH modules has a constant vi with a 5000 ms timeout value, what this script does is to make sure that the selected request utilizes Module Timeout--constant.vi no matter what the value it is inside."
            n96 = Unbundle By Name(w685) -> ("Current Selection.DQMH Lib Ref"=w683:refnum<vi>, "Current Selection.VI Ref"=w684:refnum<vi>)
            n97 = call "Script Request and Wait For Reply Restore Timeout.vi"("error in"=w687, "VI Ref"=w684, "DQMH Lib Ref"=w683) -> ("error out"=w686:errorcluster)  [unwired: 8 in]
          }
          frame "Open Front Panel" {
            # "User Selection 'Open Front Panel'"
            n98 = Unbundle By Name(w691) -> ("Current Selection.VI Ref"=w690:refnum<vi>)
            n99 = invoke class="VI" method="FP.Open"(reference=w690, error in=w693, "Activate"=TRUE ("Activate?"), "State"=T31."Standard") -> (error out=w692:errorcluster)  [unwired: 1 in, 4 out]
          }
          frame "Module ID Update" {
            # "Module ID Control has value change"
            n100 = Variant To Data(error in=w700, type=0 ("Module ID"), Variant=w697) -> (data=w695:i32, error out=w699:errorcluster)
            n101 = Bundle By Name(cluster=w698, "Module ID"=w695) -> (w696:T5)
          }
          frame "Expand or Close" {
            # "Expand or Close DQMH Tree control"
            n102 = Variant To Data(error in=w707, type=T17 {"Expand?"=FALSE} ("Expand or Close Argument"), Variant=w704) -> (data=w702:T17, error out=w706:errorcluster)
            n103 = Unbundle By Name(w702) -> ("Expand?"=w701:bool)
            n104 = invoke on="Modules Tree" class="Tree (strict)" method="Open/Close.Open/Close All"("Open"=w701) -> ()  [unwired: 3 in, 4 out]
          }
          frame "Launch DQMH Scripting Tools" {
            # "Launch the DQMH Scripting Tools"
            n105 = Variant To Data(error in=w720, type=T13 {"Scripting Tool"=enum."Create New DQMH Event"} ("Launch DQMH Scripting Tools Argument"), Variant=w717) -> (data=w715:T13, error out=w719:errorcluster)
            n106 = Unbundle By Name(w715) -> ("Scripting Tool"=w710:T14)
            n107 = Unbundle By Name(w709) -> ("DQMH Scan Results.Project References.Project Name"=w713:string, "DQMH Scan Results.Project References.App Ref"=w714:refnum<vi>, "Current Selection.DQMH Lib Ref"=w708:refnum<vi>)
            n108 = Format Into String(format string="DQMH Tool: %s being executed ", w710) -> (resulting string=w712:string)  [unwired: 2 in, 1 out]
            n109 = call "Status Updated.vi"("Status"=w712) -> ()  [unwired: 10 in, 1 out]
            n110 = call "Launch DQMH Tools by menu.vi"("Project"=w713, "Application Instance"=w714, "error in"=w719, "Module Ref"=w708, "DQMH Tools"=w710) -> ("error out"=w718:errorcluster)  [unwired: 6 in]
          }
          frame "-------PANTHER---------" {
          }
          frame "Set App Theme" {
            # "Set Panther Dashboard Theme"
            n111 = Variant To Data(error in=w732, type=T22 {"Theme"=FALSE} ("Set App Theme Argument"), Variant=w728) -> (data=w726:T22, error out=w731:errorcluster)
            n112 = Unbundle By Name(w726) -> ("Theme"=w723:bool)
            n113 = control-ref of="This VI"() -> (w725:refnum<vi>)
            n114 = Bundle By Name(cluster=w729, "Theme"=w723) -> (w724:T5)
            n115 = call "Set Theme.vi"("Dark?"=w723, "VI in"=w725) -> ()  [unwired: 10 in]
            n116 = call "Theme Updated.vi"("Theme"=w723) -> ()  [unwired: 10 in, 1 out]
            n117 = call "Save Theme in config.vi"("error in"=w731, "Theme"=w723) -> ("error out"=w730:errorcluster)  [unwired: 9 in]
          }
          frame "Show About" {
            # "Show About project"
            n118 = Variant To Data(error in=w741, type=T23 {"Boolean"=FALSE} ("Show About Argument"), Variant=w735) -> (error out=w738:errorcluster)  [unwired: 1 out]
            n119 = control-ref of="This VI"() -> (w733:refnum<vi>)
            n120 = call "Hide VI Panel.vi"("error in (no error)"=w738, "VI"=w733) -> ("error out"=w740:errorcluster)  [unwired: 9 in]
            n121 = call "About Panther Dashboard.vi"("error in"=w740) -> ("error out"=w739:errorcluster)  [unwired: 10 in]
            n122 = call "Open VI Panel.vi"("error in (no error)"=w739, "VI"=w733) -> ("error out"=w737:errorcluster)  [unwired: 9 in]
          }
          frame "Update Module ID" {
            # "Update the Current Module ID"
            n123 = Variant To Data(error in=w749, type=T24 {"New ID"=-1} ("Update Module ID Argument"), Variant=w746) -> (data=w744:T24, error out=w748:errorcluster)
            n124 = Unbundle By Name(w744) -> ("New ID"=w742:i32)
            n125 = Bundle By Name(cluster=w747, "Module ID"=w742) -> (w743:T5)
          }
          frame "Tree DQMH Selection" {
            # "There is a new selection of the DQMH Tree list, need to search and update indicators acordanly."
            n126 = Unbundle By Name(w759) -> ("Maps.Tree Map"=w758:T7, "Maps.References Map"=w757:map{string, refnum<vi>}, "DQMH Scan Results"=w756:T8)
            n127 = Variant To Data(error in=w764, type=T16 {"Tree DQMH Sel"=""} ("Tree DQMH Selection Argument"), Variant=w762) -> (data=w760:T16, error out=w763:errorcluster)
            n128 = Unbundle By Name(w760) -> ("Tree DQMH Sel"=w753:string)
            n129 = call "Get List Information.vi"("List Selection"=w753, "DQMH Scan Info"=w756, "References Map"=w757, "Tree Map"=w758) -> ("Broadcast?"=w752:bool, "Vi out"=w751:refnum<vi>, "Module type"=w750:T9, "DQMH Lib"=w754:refnum<vi>)  [unwired: 4 in]
            n130 = Bundle By Name(cluster=w759, "Current Selection.DQMH Lib Ref"=w754, "Module type"=w750, "Current Selection.VI Ref"=w751, "Broadcast?"=w752) -> (w755:T5)
          }
          frame "-------PROJECT----------" {
          }
          frame "Open Project Folder" {
            n131 = Unbundle By Name(w769) -> ("DQMH Scan Results.Project References.Project Ref"=w768:refnum<vi>)
            n132 = property class="Project"(reference=w768) -> ("Path"=w767:path)  [unwired: 1 in, 2 out]
            n133 = call "Open File on Disk.vi"("error in"=w771, "file or directory path"=w767) -> ("error out"=w770:errorcluster)  [unwired: 9 in]
          }
          frame "Show Project DQMH Info" {
            n134 = Unbundle By Name(w778) -> ("DQMH Scan Results.All Modules type"=w772:T9[], "Theme"=w775:bool, "DQMH Scan Results.Project References.App Ref"=w777:refnum<vi>, "DQMH Scan Results.All DQMH Modules Refs"=w773:refnum<vi>[])
            n135 = call "Status Updated.vi"("Status"="Getting Project info") -> ("error out"=w779:errorcluster)  [unwired: 10 in]
            n136 = Empty Array?(array=w773) -> (empty?=w774:bool)
            n137 = case shown="False" w774 {
              tunnel: w773 -> [w787 _]
              tunnel: w781 -> [w792 w796]
              tunnel: w777 -> [w786 _]
              tunnel: [w790 w794] -> w780
              tunnel: w775 -> [w785 _]
              tunnel: w779 -> [_ _]
              tunnel: w772 -> [w782 _]
              frame False {
                # "Project has been scanned"
                n138 = call "Script Parse Project Modules Constants.vi"("App Ref"=w786, "error in"=w792, "All DQMH Modules Refs"=w787) -> ("error out"=w791:errorcluster, "Project info Results"=w783:string[][])  [unwired: 7 in]
                n139 = call "Hide Panel.vi"("error in (no error)"=w791) -> ("error out"=w789:errorcluster)  [unwired: 10 in]
                n140 = call "Insert Module Types.vi"("All Modules types"=w782, "Project info Results In"=w783) -> ("Project info Results Out"=w784:string[][])  [unwired: 9 in]
                n141 = call "Display Project Info Results.vi"("Theme"=w785, "error in"=w789, "Project Results"=w784) -> ("error out"=w788:errorcluster)  [unwired: 8 in]
                n142 = call "Show Panel.vi"("error in (no error)"=w788) -> ("error out"=w790:errorcluster)  [unwired: 10 in]
              }
              frame True {
                n143 = invoke on="Projects" class="CmbBox" method="ObjHighlight"(error in=w796) -> (error out=w795:errorcluster)  [unwired: 2 in, 2 out]
                n144 = invoke on="Search" class="Bool" method="ObjHighlight"(error in=w795) -> (error out=w794:errorcluster)  [unwired: 2 in, 2 out]
                n145 = call "Status Updated.vi"("Status"="Please Scan your Project first") -> ()  [unwired: 10 in, 1 out]
              }
            }
          }
          frame "--------DOCUMENTATION------" {
          }
          frame "Generate Project Documentation" {
            n146 = Variant To Data(error in=w807, type=T21 {"Boolean"=FALSE} ("Generate Project Documentation Argument"), Variant=w803) -> (error out=w806:errorcluster)  [unwired: 1 out]
            n147 = Unbundle By Name(w801) -> ("DQMH Scan Results.Project References.Project Ref"=w800:refnum<vi>)
            n148 = property class="Project"(reference=w800) -> ("Path"=w799:path)  [unwired: 1 in, 2 out]
            n149 = call "Generate Documentation--dialog.vi"("Project Path"=w799) -> ("error out"=w804:errorcluster)  [unwired: 10 in]
            n150 = Merge Errors(w806, w804) -> (w805:errorcluster)
          }
          frame "Save VI Description" {
            # "Save Event Description"
            n151 = Variant To Data(error in=w817, type=T26 {"VI Description"=""} ("Save VI Description Argument"), Variant=w813) -> (data=w811:T26, error out=w816:errorcluster)
            n152 = Unbundle By Name(w811) -> ("VI Description"=w809:string)
            n153 = in-place {
              in-place-border: w809 -> [w820]
              in-place-border: [w821] -> w814
              n154 = in-place-cluster #1(w810) -> ("Current Selection.VI Ref"=w819:refnum<vi>)
              n155 = call "Save Event Description.vi"("Event Description"=w820, "Event Ref in"=w819) -> ("error out"=w821:errorcluster, "Event Ref out"=w818:refnum<vi>)  [unwired: 8 in]
              n156 = in-place-cluster #1("Current Selection.VI Ref"=w818) -> (w808:T5)
            }
            n157 = Merge Errors(w816, w814) -> (w815:errorcluster)
          }
          frame "Save Library Description" {
            # "Save Library Description"
            n158 = Variant To Data(error in=w831, type=T25 {"Library Description"=""} ("Save Library Description Argument"), Variant=w827) -> (data=w825:T25, error out=w830:errorcluster)
            n159 = Unbundle By Name(w825) -> ("Library Description"=w824:string)
            n160 = in-place {
              in-place-border: w824 -> [w835]
              in-place-border: [w837] -> w828
              n161 = in-place-cluster #2(w823) -> ("Current Selection.DQMH Lib Ref"=w836:refnum<vi>, "DQMH Scan Results"=w833:T8)
              n162 = call "Save Library Documentation.vi"("New Description"=w835, "DQMH Modules Info In"=w833, "Library in"=w836) -> ("error out"=w837:errorcluster, "DQMH Modules Info Out"=w834:T8, "Lib out"=w832:refnum<vi>)  [unwired: 6 in]
              n163 = in-place-cluster #2("Current Selection.DQMH Lib Ref"=w832, "DQMH Scan Results"=w834) -> (w822:T5)
            }
            n164 = Merge Errors(w830, w828) -> (w829:errorcluster)
          }
          frame "Open Documentation" {
            # "Open Antidoc Documentation"
            n165 = Variant To Data(error in=w849, type=T27 {"Boolean"=FALSE} ("Open Documentation Argument"), Variant=w847) -> (error out=w848:errorcluster)  [unwired: 1 out]
            n166 = Unbundle By Name(w838) -> ("DQMH Scan Results.Project References.Project Ref"=w845:refnum<vi>)
            n167 = property class="Project"(reference=w845) -> ("Path"=w844:path)  [unwired: 1 in, 2 out]
            n168 = Strip Path(path=w844) -> (stripped path=w843:path)  [unwired: 1 out]
            n169 = Build Path(base path=w843, name or relative path=path "Antidoc-Output/Project-Documentation.pdf") -> (appended path=w842:path)
            n170 = call <vilib>:"Check if File or Folder Exists.vi"("path"=w842) -> ("file or folder exists?"=w840:bool, "dup path"=w841:path)  [unwired: 8 in, 1 out]
            n171 = case shown="False" w840 {
              tunnel: w841 -> [_ w851]
              frame False {
                n172 = invoke on="Generate Antidoc" class="Bool" method="ObjHighlight"() -> ()  [unwired: 3 in, 3 out]
                n173 = call "Status Updated.vi"("Status"="No Antidoc Output has been found, please select a project and generate it first.") -> ()  [unwired: 10 in, 1 out]
              }
              frame True {
                n174 = call-poly <vilib>:"Open URL in Default Browser.vi"("path"=w851) -> ()  [unwired: 5 in, 2 out]
              }
            }
          }
          frame "Save Project Documentation" {
            n175 = Variant To Data(error in=w860, type=T28 {"Project Description"=""} ("Save Project Documentation Argument"), Variant=w857) -> (data=w855:T28, error out=w859:errorcluster)
            n176 = Unbundle By Name(w855) -> ("Project Description"=w852:string)
            n177 = Unbundle By Name(w854) -> ("DQMH Scan Results.Project References.Project Ref"=w853:refnum<vi>)
            n178 = property class="Project"(reference=w853, error in=w859, "Description"=w852) -> (error out=w858:errorcluster)  [unwired: 1 out]
          }
          frame "---Exit and Error Handling---" {
            # "Separator - The following cases handle errors and exit messages."
          }
          frame "Error" {
            # "Error - Check the error message data and respond accordingly. This message is sent by the \"Error Handler\" VIs at the end of each loop in this application."
            n179 = property on="Property Node" class="Module Admin"(reference=w864) -> ("Accessors:External Launch"=w863:bool)  [unwired: 1 in, 2 out]
            n180 = Variant To Data(error in=w872, type=errorcluster {"status"=FALSE, "code"=0, "source"=""} ("error constant"), Variant=w866) -> (data=w873:errorcluster, error out=w870:errorcluster)
            n181 = call "Error Reported.vi"("Error"=w873) -> ()  [unwired: 10 in, 1 out]
            n182 = case shown="True" w863 {
              tunnel: [w878 _] -> w869
              tunnel: w865 -> [w876 _]
              tunnel: w873 -> [w877 _]
              frame False {
                # "If the module is running standalone, then pop up an error dialog and call the \"Exit\" message."
                n183 = call <vilib>:"Simple Error Handler.vi"("error in (no error)"=w877) -> ()  [unwired: 4 in, 5 out]
                n184 = call-poly <vilib>:"Delacor_lib_QMH_Enqueue Message (poly).vi"("Priority Message? (F)"=TRUE, "Message"="Exit", "Message Queue in"=w876) -> ("error out"=w878:errorcluster)  [unwired: 7 in, 1 out]
              }
              frame True {
                # "If the module was launched externally, calling the Error Reported broadcast VI is the only action performed by the \"Error\" message. The module's caller can then process the error appropriately."
              }
            }
            n185 = Merge Errors(w870, w869) -> (w868:errorcluster)
            n186 = local write "error out"(w868) -> ()
          }
          frame "Exit" {
            w885 = 91  # 91: not all Exit messages will have an argument
            w887 = TRUE  # Stop the VI
            # "Release the message queue reference"
            # "Exit - Exit the application."
            n187 = Variant To Data(error in=w894, type=T20 {"Origin"="", "Exit via Stop Module Req?"=FALSE, "Wait for Module to stop?"=FALSE} ("Stop Argument"), Variant=w886) -> (data=w883:T20, error out=w890:errorcluster)
            n188 = call <vilib>:"Clear Errors.vi"("error in (no error)"=w890, "specific error code to clear (0: all)"=w885) -> ("error out"=w893:errorcluster)  [unwired: 4 in, 1 out]
            n189 = control-ref of="This VI"() -> (w882:refnum<vi>)
            n190 = invoke on="Modules Tree" class="Tree (strict)" method="Edit Tree Items.Delete"() -> ()  [unwired: 5 in, 5 out]
            n191 = call-dynamic "Delacor_lib_QMH_Release Message Queue.vi"("error in"=w893, "Message Queue"=w888) -> ("error out"=w892:errorcluster)  [unwired: 9 in]
            n192 = call "Handle Exit.vi"("Stop Argument"=w883, "Admin in"=w881, "VI reference"=w882) -> ("error out"=w889:errorcluster)  [unwired: 7 in, 1 out]
            n193 = call "Close vi references.vi"("Data Cluster"=w880) -> ()  [unwired: 10 in, 1 out]
            n194 = Merge Errors(w892, w889) -> (w891:errorcluster)
            n195 = call "Error Reported.vi"("Error"=w891) -> ()  [unwired: 10 in, 1 out]
            n196 = call "Stop Module.vi"("Origin"="Panther Dahsboard Stopped") -> ()  [unwired: 10 in, 1 out]
          }
          frame Default {
            # "'Default' case only runs if there is a message that isn't defined in any of the other cases.  Output a programming error."
            n197 = call "Module Name--constant.vi"() -> ("Module Name"=w895:string)  [unwired: 11 in]
            n198 = xnode ("Error Ring")("parameter 0"=w896, "parameter 1"=w895) -> ("error out"=w900:errorcluster)
            n199 = Merge Errors(w898, w900) -> (w899:errorcluster)
          }
          frame "Save Module Spec" {
            # "Save current module tree specification to disk."
            n200 = Variant To Data(error in=w915, type=T29 {"Boolean"=FALSE} ("Save Module Spec Argument"), Variant=w913) -> (error out=w914:errorcluster)  [unwired: 1 out]
            n201 = control-ref of="Modules Tree"() -> (w910:refnum<vi>)
            n202 = property class="Tree (strict)"(reference=w910) -> ("All Tags"=w909:string[])  [unwired: 1 in, 2 out]
            n203 = Write to Text File(text=w909) -> ()  [unwired: 3 in, 3 out]
          }
        }
        n204 = call-dynamic "Delacor_lib_QMH_Error Handler - Message Handling Loop.vi"("error in"=w475, "Ignore Errors (Runtime)"=w463, "Message Queue in"=w465) -> ("dup error in"=w472:errorcluster)  [unwired: 7 in, 1 out]
      }
      n205 = while {
        tunnel: w31 -> [w143]
        shift-right: [w145] -> w37
        shift-left: w35 -> [w146]
        tunnel: [w147] -> w40
        shift-right: [w141] -> _
        shift-left: w30 -> [w140]
        shift-right: [w139] -> _
        shift-left: Selection_Type--enum."Public API" ("Selection type") -> [w138]
        stop <- w144 stop-if-true
        # "Event Handling Loop"
        n206 = event "DQMH_EVENT_MAIN" shown="[6] \"Modules Tree\": Value Change" {
          selector: w146 -> [_ _ _ _ _ _ _ _ _ _ _ _ _ _ _ _ _ _ _ _ _ _ _ _ _ _ _ _ _ _ _ _ _ _ _ _ _ _]
          dyn-events: [_ _ _ _ _ _ _ _ _ _ _ _ _ _ _ _ _ _ _ _ _ _ _ _ _ _ _ _ _ _ _ _ _ _ _ _ _ _] -> w145
          timeout: 3000 -> [_ _ _ _ _ _ _ _ _ _ _ _ _ _ _ _ _ _ _ _ _ _ _ _ _ _ _ _ _ _ _ _ _ _ _ _ _ _]
          tunnel: [_ _ _ _ _ _ _ _ _ _ _ _ _ _ _ _ _ _ _ TRUE ("Discard?") _ _ _ _ _ _ _ _ _ _ _ _ _ _ _ _ _ _] -> w144
          tunnel: w143 -> [w149 _ _ w182 w194 w199 w218 _ w227 _ w241 w251 w259 _ _ w275 w284 _ _ w319 w328 _ w339 w347 w355 w363 w371 w379 w387 w395 w403 w411 w419 w427 w435 w443 w452 w460]
          tunnel: [w158 w173 w178 w183 w195 w200 w219 w224 w230 w238 w244 w252 w260 w264 _ w276 w285 _ w310 w322 w330 w334 w342 w350 w358 w366 w374 w382 w390 w398 w406 w414 w422 w430 w438 w446 w447 w456] -> w148
          tunnel: [w157 w172 w177 w180 w191 w197 w214 w220 w229 w237 w243 w246 w255 w262 w266 w270 w282 w298 w309 w312 w325 w333 w341 w349 w357 w365 w373 w381 w389 w397 w405 w413 w421 w429 w437 w445 w454 w462] -> w141
          tunnel: w140 -> [w157 w172 w177 w180 w191 w197 _ w220 w229 w237 w243 w246 w255 w262 w266 w270 w282 w298 w309 w312 w325 w333 w341 w349 w357 w365 w373 w381 w389 w397 w405 w413 w421 w429 w437 w445 w454 w462]
          tunnel: [w156 w171 w176 w179 w190 w196 w212 w222 w228 w236 w242 w245 w254 w261 w265 w269 w281 w297 w308 w311 w324 w332 w340 w348 w356 w364 w372 w380 w388 w396 w404 w412 w420 w428 w436 w444 w453 w461] -> w139
          tunnel: w138 -> [w156 w171 w176 _ w190 w196 _ w222 w228 w236 w242 w245 w254 w261 w265 w269 w281 w297 w308 w311 w324 w332 w340 w348 w356 w364 w372 w380 w388 w396 w404 w412 w420 w428 w436 w444 w453 w461]
          event "Add Event", "Remove Event", "Convert Event", "Rename Event", "Add New Module", "Rename Module", "Validate Module", "Create Module Template", "Add Unit Test Module", "Create RT Tester Module", "Add Helper Loop to Module": Value Change {
            n207 = event-data() -> ("CtlRef"=w154:refnum<vi>)  [unwired: 1 in]
            n208 = property class="Bool"(reference=w154) -> ("Label.Text"=w155:string)  [unwired: 1 in, 2 out]
            n209 = case shown="\"Add Helper Loop to Module\"" w155 {
              tunnel: [DQMH_Tools_Menu--enum."Create New DQMH Event" ("DQMH Tools") DQMH_Tools_Menu--enum."Convert DQMH Event" ("DQMH Tools") DQMH_Tools_Menu--enum."Remove DQMH Event" ("DQMH Tools") DQMH_Tools_Menu--enum."Rename DQMH Event" ("DQMH Tools") DQMH_Tools_Menu--enum."Add New DQMH Module" ("DQMH Tools") DQMH_Tools_Menu--enum."Rename DQMH Module" ("DQMH Tools") DQMH_Tools_Menu--enum."Validate DQMH Module" ("DQMH Tools") DQMH_Tools_Menu--enum."Create RT Tester" ("DQMH Tools") DQMH_Tools_Menu--enum."New DQMH  Unit Test" ("DQMH Tools") DQMH_Tools_Menu--enum."Create DQMH Module Template" ("DQMH Tools") DQMH_Tools_Menu--enum."Add Helper Loop to DQMH Module" ("DQMH Tools")] -> w150
              frame "Add Event", Default {
              }
              frame "Convert Event" {
              }
              frame "Remove Event" {
              }
              frame "Rename Event" {
              }
              frame "Add New Module" {
              }
              frame "Rename Module" {
              }
              frame "Validate Module" {
              }
              frame "Create RT Tester Module" {
              }
              frame "Add Unit Test Module" {
              }
              frame "Create Module Template" {
              }
              frame "Add Helper Loop to Module" {
              }
            }
            n210 = Bundle(cluster=T13 {"Scripting Tool"=enum."Create New DQMH Event"} ("Launch DQMH Scripting Tools Argument"), "Scripting Tool"=w150) -> (w153:T13)
            n211 = call-poly <vilib>:"Delacor_lib_QMH_Enqueue Message (poly).vi"("Message Data"=w153, "Message"="Launch DQMH Scripting Tools", "Message Queue in"=w149) -> ("error out"=w158:errorcluster)  [unwired: 7 in, 1 out]
          }
          event "Context Help Panther": Value Change {
            # "Open Documentation DQMH Module"
            n212 = event-data() -> ()  [unwired: 1 in, 1 out]
            n213 = case shown="True" "Context Help Panther" {
              tunnel: [w174 w175] -> w173
              frame False {
                n214 = call "Hide Panel.vi"() -> ("error out"=w174:errorcluster)  [unwired: 11 in]
              }
              frame True {
                n215 = call "Show Panel.vi"() -> ("error out"=w175:errorcluster)  [unwired: 11 in]
              }
            }
          }
          event User Event {
            # "We wait for the Context help module to init to send a request to refresh \npanther Dashboard Broadcasts, we need this module to be\nlistening Panther Dashboard broadcasts"
            n216 = event-data() -> ()  [unwired: 1 in, 1 out]
            n217 = call "Refresh Panther Dashboard Broadcasts.vi"() -> ("error out"=w178:errorcluster)  [unwired: 11 in]
          }
          event "Modules Tree": Double Click {
            # "User double click an element on the tree control, we check if it is an event to find its frame on the corresponding DQMH module, we also check if it is a broadcast to find where is being triggered"
            n218 = event-data() -> ("Tag"=w181:string)  [unwired: 1 in]
            n219 = call "Validate if event is selected.vi"("Tree Selection"=w181) -> ("Selection type"=w179:T4)  [unwired: 10 in]
            n220 = case shown="\"Module\"" w179 {
              tunnel: [w186 _ w189] -> w183
              tunnel: w182 -> [w185 _ w188]
              frame "Module" {
                # "Selection is a module"
                n221 = call-poly <vilib>:"Delacor_lib_QMH_Enqueue Message (poly).vi"("Message"="Find Module in project", "Message Queue in"=w185) -> ("error out"=w186:errorcluster)  [unwired: 8 in, 1 out]
              }
              frame "Public API" {
              }
              frame "Broadcast".."Request and Wait for Reply" {
                # "Selection is an Event vi?"
                n222 = call-poly <vilib>:"Delacor_lib_QMH_Enqueue Message (poly).vi"("Message"="Locate Event on Main", "Message Queue in"=w188) -> ("error out"=w189:errorcluster)  [unwired: 8 in, 1 out]
              }
            }
          }
          event "Modules Tree": Drag Starting? {
            # "Drag current selection to user destination"
            n223 = event-data() -> ()  [unwired: 1 in, 1 out]
            n224 = call-poly <vilib>:"Delacor_lib_QMH_Enqueue Message (poly).vi"("Message"="Drag VI", "Message Queue in"=w194) -> ("error out"=w195:errorcluster)  [unwired: 8 in, 1 out]
            n225 = event-data("Discard?"=TRUE) -> ()  [unwired: 1 in, 1 out]
          }
          event "Modules Tree": Shortcut Menu Selection (User) {
            # "User selects something from the Right Click Shortcut Menu"
            n226 = event-data() -> ("ItemTag"=w198:string)  [unwired: 1 in]
            n227 = case shown="Default" w198 {
              selector: w198 -> [w203 w209]
              tunnel: w199 -> [w207 w210]
              tunnel: [w208 w211] -> w200
              frame "-Run: Hide Panel", "-Run: Show Diagram", "-Run: Show Panel", "-Run: Stop Module" {
                n228 = Match Pattern(string=w203, regular expression="-Run: ") -> (after substring=w202:string)  [unwired: 1 in, 3 out]
                n229 = Bundle(cluster=T15 {"Event Name"=""} ("Execute Default Event Request Argument"), "Event Name"=w202) -> (w205:T15)
                n230 = call-poly <vilib>:"Delacor_lib_QMH_Enqueue Message (poly).vi"("Message Data"=w205, "Message"="Execute Default Event Request", "Message Queue in"=w207) -> ("error out"=w208:errorcluster)  [unwired: 7 in, 1 out]
              }
              frame Default {
                n231 = call-poly <vilib>:"Delacor_lib_QMH_Enqueue Message (poly).vi"("Message"=w209, "Message Queue in"=w210) -> ("error out"=w211:errorcluster)  [unwired: 8 in, 1 out]
              }
            }
          }
          event "Modules Tree": Value Change {
            w214 = TRUE  # Tree valid Selection
            # "The user selected an item on the tree control"
            n232 = event-data() -> ()  [unwired: 1 in, 1 out]
            n233 = Bundle(cluster=T16 {"Tree DQMH Sel"=""} ("Tree DQMH Selection Argument"), "Tree DQMH Sel"="Modules Tree") -> (w215:T16)
            n234 = call "Validate if event is selected.vi"("Tree Selection"="Modules Tree") -> ("Selection type"=w212:T4)  [unwired: 10 in]
            n235 = call-poly <vilib>:"Delacor_lib_QMH_Enqueue Message (poly).vi"("Message Data"=w215, "Message"="Tree DQMH Selection", "Message Queue in"=w218) -> ("error out"=w219:errorcluster)  [unwired: 7 in, 1 out]
          }
          event "Modules Tree": Shortcut Menu Activation? {
            # "This is wher the shorcut menu is filled, only after the user select a module"
            n236 = event-data() -> ("MenuRef"=w223:refnum<k9>)  [unwired: 1 in]
            n237 = call "Create Tree Shortcut Menu.vi"("Selection type"=w222, "Menu in"=w223) -> ("error out"=w224:errorcluster)  [unwired: 9 in]
            n238 = Not(x=w220) -> (.not. x?=w221:bool)
            n239 = event-data("Discard?"=w221) -> ()  [unwired: 1 in, 1 out]
          }
          event "Projects": Value Change {
            n240 = event-data() -> ()  [unwired: 1 in, 1 out]
            n241 = call-poly <vilib>:"Delacor_lib_QMH_Enqueue Message (poly).vi"("Message Data"="Projects", "Message"="Refresh Targets", "Message Queue in"=w227) -> ("error out"=w230:errorcluster)  [unwired: 7 in, 1 out]
          }
          event "Projects": Shortcut Menu Activation? {
            n242 = event-data() -> ("MenuRef"=w235:refnum<k9>)  [unwired: 1 in]
            n243 = Delete Menu Items(9:w235) -> (0:w239:errorcluster, 3:w234:refnum<k9>)  [unwired: 3 in]
            n244 = Insert Menu Items(6:w239, 8:string[] ["Open Project Folder", "Show Project DQMH Info"] ("item names"), 9:w234) -> (0:w238:errorcluster)  [unwired: 3 in, 2 out]
            n245 = local read "Projects"() -> (w232:string)
            n246 = Empty String/Path?(string/path=w232) -> (empty?=w231:bool)
            n247 = event-data("Discard?"=w231) -> ()  [unwired: 1 in, 1 out]
          }
          event "Projects": Shortcut Menu Selection (User) {
            n248 = event-data() -> ("ItemTag"=w240:string)  [unwired: 1 in]
            n249 = call-poly <vilib>:"Delacor_lib_QMH_Enqueue Message (poly).vi"("Message"=w240, "Message Queue in"=w241) -> ("error out"=w244:errorcluster)  [unwired: 8 in, 1 out]
          }
          event User Event {
            # "Another Module called the \"Expand or Close\" API Method."
            n250 = event-data() -> ("Expand?"=w247:bool)  [unwired: 1 in]
            n251 = Bundle(cluster=T17 {"Expand?"=FALSE} ("Expand or Close Argument"), "Expand?"=w247) -> (w248:T17)
            n252 = call-poly <vilib>:"Delacor_lib_QMH_Enqueue Message (poly).vi"("Message Data"=w248, "Message"="Expand or Close", "Message Queue in"=w251) -> ("error out"=w252:errorcluster)  [unwired: 7 in, 1 out]
          }
          event "Expand Results": Value Change {
            # "Another Module called the \"Expand or Close\" API Method."
            n253 = event-data() -> ()  [unwired: 1 in, 2 out]
            n254 = Bundle(cluster=T17 {"Expand?"=FALSE} ("Expand or Close Argument"), "Expand?"="Expand Results") -> (w256:T17)
            n255 = call-poly <vilib>:"Delacor_lib_QMH_Enqueue Message (poly).vi"("Message Data"=w256, "Message"="Expand or Close", "Message Queue in"=w259) -> ("error out"=w260:errorcluster)  [unwired: 7 in, 1 out]
          }
          event User Event {
            # "Another Module called the \"Get Module Execution Status\" API Method."
            n256 = event-data() -> ()  [unwired: 1 in, 1 out]
            n257 = call "Update Module Execution Status.vi"("Running?"=TRUE) -> ("error out"=w264:errorcluster)  [unwired: 10 in]
          }
          event User Event {
            # "Hide the panel of this VI, and send a status updated message to let listeners know."
            # "Another Module called the \"Hide Panel\" API Method."
            n258 = event-data() -> ()  [unwired: 1 in, 1 out]
            n259 = control-ref of="This VI"() -> (w267:refnum<vi>)
            n260 = call "Hide VI Panel.vi"("VI"=w267) -> ()  [unwired: 10 in, 1 out]
          }
          event User Event {
            # "Another Module called the \"Scan DQMH Modules\" API Method."
            n261 = event-data() -> ("Include Dependencies"=w271:bool, "Target"=w268:string)  [unwired: 1 in, 1 out]
            n262 = Bundle(cluster=T18 {"Include Dependencies"=FALSE, "Scan All"=FALSE, "Project"="", "Target"=""} ("Scan DQMH Modules Argument"), "Include Dependencies"=w271, "Project"=w268) -> (w272:T18)  [unwired: 2 in]
            n263 = call-poly <vilib>:"Delacor_lib_QMH_Enqueue Message (poly).vi"("Message Data"=w272, "Message"="Scan DQMH Modules", "Message Queue in"=w275) -> ("error out"=w276:errorcluster)  [unwired: 7 in, 1 out]
          }
          event "Search": Value Change {
            # "#via_ignore Unwired Event Nodes"
            # "Another Module called the \"Scan DQMH Modules\" API Method."
            n264 = event-data() -> ()  [unwired: 1 in, 1 out]
            n265 = local read "Projects"() -> (w280:string)
            n266 = Empty String/Path?(string/path="Targets") -> (empty?=w278:bool)
            n267 = global write "Panther Dashboard--global.vi" "Target"("Targets") -> ()
            n268 = Empty String/Path?(string/path=w280) -> (empty?=w283:bool)
            n269 = Or(x=w283, y=w278) -> (x .or. y?=w279:bool)
            n270 = case shown="False" w279 {
              tunnel: [w294 _] -> w285
              tunnel: w284 -> [w293 _]
              tunnel: w280 -> [w287 _]
              tunnel: "Targets" -> [w288 _]
              frame False {
                n271 = Bundle(cluster=T18 {"Include Dependencies"=FALSE, "Scan All"=FALSE, "Project"="", "Target"=""} ("Scan DQMH Modules Argument"), "Include Dependencies"="Include Dependencies", "Scan All"="Scan All", "Project"=w287, "Target"=w288) -> (w290:T18)
                n272 = call-poly <vilib>:"Delacor_lib_QMH_Enqueue Message (poly).vi"("Message Data"=w290, "Message"="Scan DQMH Modules", "Message Queue in"=w293) -> ("error out"=w294:errorcluster)  [unwired: 7 in, 1 out]
              }
              frame True {
                n273 = invoke on="Projects" class="CmbBox" method="ObjHighlight"() -> (error out=w296:errorcluster)  [unwired: 3 in, 2 out]
                n274 = invoke on="Targets" class="CmbBox" method="ObjHighlight"(error in=w296) -> ()  [unwired: 2 in, 3 out]
                n275 = call "Status Updated.vi"("Status"="Scanning requires a project and an target please make the selection.\n") -> ()  [unwired: 10 in, 1 out]
              }
            }
          }
          event User Event {
            # "Another Module called the \"Show Diagram\" API Method. This event is used for debugging."
            n276 = event-data() -> ()  [unwired: 1 in, 1 out]
            n277 = disable-structure shown="RUN_TIME_ENGINE==False" {
              frame condition #0 (active) {
                # "functionality not available in exe"
                n278 = invoke on="Invoke Node" class="VI" method="Lock State.Get"() -> (error out=w304:errorcluster, "Get Lock State"=w303:T19, "pwd in cache"=w300:bool)  [unwired: 4 in, 1 out]
                n279 = Equal?(x=T19."Password-protected", y=w303) -> (x = y?=w301:bool)
                n280 = Compound Arithmetic op=AND(w301, invert w300) -> (w299:bool)
                n281 = case shown="False" w299 {
                  tunnel: w304 -> [w306 _]
                  frame False {
                    n282 = property on="Property Node" class="VI"(error in=w306, "BDWin.Open"=TRUE ("Block Diagram Window:Open")) -> ()  [unwired: 1 in, 2 out]
                  }
                  frame True {
                    # "Password-protected VI, and the password is not in the cache. Do not show the diagram."
                  }
                }
              }
              frame condition #1 {
              }
            }
          }
          event User Event {
            # "Show the panel of this VI, and send a status updated message to let listeners know."
            # "Another Module called the \"Show Panel\" API Method."
            n283 = event-data() -> ()  [unwired: 1 in, 1 out]
            n284 = control-ref of="This VI"() -> (w307:refnum<vi>)
            n285 = call "Open VI Panel.vi"("VI"=w307) -> ()  [unwired: 10 in, 1 out]
            n286 = call "Register controls Mouse Enter.vi"() -> ("error out"=w310:errorcluster)  [unwired: 11 in]
          }
          event User Event {
            # "The Stop Module Event can get fired from the Exit message in the MHL. The queue gets destroyed in that case. If the queue no longer exists, the Enqueue Exit as a priority message will return error 1. It is safe to ignore, because the module is already exiting."
            # "Another Module called the \"Stop Module\" API Method  or the Message Handling Loop below."
            n287 = event-data() -> ("Exit via Stop Module Req?"=w315:bool, "Wait for Module to stop?"=w314:bool)  [unwired: 1 in]
            n288 = Bundle By Name(cluster=T20 {"Origin"="", "Exit via Stop Module Req?"=FALSE, "Wait for Module to stop?"=FALSE} ("Stop Argument"), "Exit via Stop Module Req?"=w315, "Wait for Module to stop?"=w314) -> (w313:T20)
            n289 = call-poly <vilib>:"Delacor_lib_QMH_Enqueue Message (poly).vi"("Priority Message? (F)"=TRUE, "Message Data"=w313, "Message"="Exit", "Message Queue in"=w319) -> ("error out"=w323:errorcluster)  [unwired: 6 in, 1 out]
            n290 = call <vilib>:"Clear Errors.vi"("error in (no error)"=w323, "specific error code to clear (0: all)"=1) -> ("error out"=w322:errorcluster)  [unwired: 4 in, 1 out]
          }
          event Panel Close? {
            w329 = TRUE  # Discard the event, the MHL is responsible for closing and stopping this VI.
            # "Hide the panel or send the 'Exit' message if the user clicks the 'X' on the module main VI panel."
            n291 = event-data() -> ()  [unwired: 1 in, 1 out]
            n292 = call-poly <vilib>:"Delacor_lib_QMH_Enqueue Message (poly).vi"("Priority Message? (F)"=TRUE, "Message"="Exit", "Message Queue in"=w328) -> ("error out"=w330:errorcluster)  [unwired: 7 in, 1 out]
            n293 = event-data ("Event Filter Node")("Discard?"=w329) -> ()  [unwired: 1 in, 1 out]
          }
          event Timeout {
            w331 = FALSE  # Init?
            n294 = event-data() -> ()  [unwired: 1 in, 1 out]
            n295 = call "Scan For App Projects.vi"("Init?"=w331) -> ("error out"=w334:errorcluster)  [unwired: 10 in]
          }
          event User Event {
            # "Another Module called the \"Launch DQMH Scripting Tools\" API Method."
            n296 = event-data() -> ("Scripting Tool"=w335:T14)  [unwired: 1 in]
            n297 = Bundle(cluster=T13 {"Scripting Tool"=enum."Create New DQMH Event"} ("Launch DQMH Scripting Tools Argument"), "Scripting Tool"=w335) -> (w336:T13)
            n298 = call-poly <vilib>:"Delacor_lib_QMH_Enqueue Message (poly).vi"("Message Data"=w336, "Message"="Launch DQMH Scripting Tools", "Message Queue in"=w339) -> ("error out"=w342:errorcluster)  [unwired: 7 in, 1 out]
          }
          event User Event {
            # "Another Module called the \"Generate Project Documentation\" API Method."
            n299 = event-data() -> ("Boolean"=w343:bool)  [unwired: 1 in]
            n300 = Bundle(cluster=T21 {"Boolean"=FALSE} ("Generate Project Documentation Argument"), "Boolean"=w343) -> (w344:T21)
            n301 = call-poly <vilib>:"Delacor_lib_QMH_Enqueue Message (poly).vi"("Message Data"=w344, "Message"="Generate Project Documentation", "Message Queue in"=w347) -> ("error out"=w350:errorcluster)  [unwired: 7 in, 1 out]
          }
          event "Generate Antidoc": Value Change {
            # "Another Module called the \"Generate Project Documentation\" API Method."
            n302 = event-data() -> ()  [unwired: 1 in, 1 out]
            n303 = Bundle(cluster=T21 {"Boolean"=FALSE} ("Generate Project Documentation Argument"), "Boolean"="Generate Antidoc") -> (w352:T21)
            n304 = call-poly <vilib>:"Delacor_lib_QMH_Enqueue Message (poly).vi"("Message Data"=w352, "Message"="Generate Project Documentation", "Message Queue in"=w355) -> ("error out"=w358:errorcluster)  [unwired: 7 in, 1 out]
          }
          event User Event {
            # "Another Module called the \"Set App Theme\" API Method."
            n305 = event-data() -> ("Theme"=w359:bool)  [unwired: 1 in]
            n306 = Bundle(cluster=T22 {"Theme"=FALSE} ("Set App Theme Argument"), "Theme"=w359) -> (w360:T22)
            n307 = call-poly <vilib>:"Delacor_lib_QMH_Enqueue Message (poly).vi"("Message Data"=w360, "Message"="Set App Theme", "Message Queue in"=w363) -> ("error out"=w366:errorcluster)  [unwired: 7 in, 1 out]
          }
          event "Theme Panther": Value Change {
            # "Another Module called the \"Set App Theme\" API Method."
            n308 = event-data() -> ()  [unwired: 1 in, 1 out]
            n309 = Bundle(cluster=T22 {"Theme"=FALSE} ("Set App Theme Argument"), "Theme"="Theme Panther") -> (w368:T22)
            n310 = call-poly <vilib>:"Delacor_lib_QMH_Enqueue Message (poly).vi"("Message Data"=w368, "Message"="Set App Theme", "Message Queue in"=w371) -> ("error out"=w374:errorcluster)  [unwired: 7 in, 1 out]
          }
          event User Event {
            # "Another Module called the \"Show About\" API Method."
            n311 = event-data() -> ("Boolean"=w375:bool)  [unwired: 1 in]
            n312 = Bundle(cluster=T23 {"Boolean"=FALSE} ("Show About Argument"), "Boolean"=w375) -> (w376:T23)
            n313 = call-poly <vilib>:"Delacor_lib_QMH_Enqueue Message (poly).vi"("Message Data"=w376, "Message"="Show About", "Message Queue in"=w379) -> ("error out"=w382:errorcluster)  [unwired: 7 in, 1 out]
          }
          event "About Panther": Value Change {
            # "Another Module called the \"Show About\" API Method."
            n314 = event-data() -> ()  [unwired: 1 in, 1 out]
            n315 = Bundle(cluster=T23 {"Boolean"=FALSE} ("Show About Argument"), "Boolean"="About Panther") -> (w384:T23)
            n316 = call-poly <vilib>:"Delacor_lib_QMH_Enqueue Message (poly).vi"("Message Data"=w384, "Message"="Show About", "Message Queue in"=w387) -> ("error out"=w390:errorcluster)  [unwired: 7 in, 1 out]
          }
          event User Event {
            # "Another Module called the \"Update Module ID\" API Method."
            n317 = event-data() -> ("New ID"=w391:i32)  [unwired: 1 in]
            n318 = Bundle(cluster=T24 {"New ID"=-1} ("Update Module ID Argument"), "New ID"=w391) -> (w392:T24)
            n319 = call-poly <vilib>:"Delacor_lib_QMH_Enqueue Message (poly).vi"("Message Data"=w392, "Message"="Update Module ID", "Message Queue in"=w395) -> ("error out"=w398:errorcluster)  [unwired: 7 in, 1 out]
          }
          event "Module ID": Value Change {
            # "Another Module called the \"Update Module ID\" API Method."
            n320 = event-data() -> ()  [unwired: 1 in, 1 out]
            n321 = Bundle(cluster=T24 {"New ID"=-1} ("Update Module ID Argument"), "New ID"="Module ID") -> (w400:T24)
            n322 = call-poly <vilib>:"Delacor_lib_QMH_Enqueue Message (poly).vi"("Message Data"=w400, "Message"="Update Module ID", "Message Queue in"=w403) -> ("error out"=w406:errorcluster)  [unwired: 7 in, 1 out]
          }
          event User Event {
            # "Another Module called the \"Save Library Description\" API Method."
            n323 = event-data() -> ("Library Description"=w407:string)  [unwired: 1 in]
            n324 = Bundle(cluster=T25 {"Library Description"=""} ("Save Library Description Argument"), "Library Description"=w407) -> (w408:T25)
            n325 = call-poly <vilib>:"Delacor_lib_QMH_Enqueue Message (poly).vi"("Message Data"=w408, "Message"="Save Library Description", "Message Queue in"=w411) -> ("error out"=w414:errorcluster)  [unwired: 7 in, 1 out]
          }
          event User Event {
            # "Another Module called the \"Save VI Description\" API Method."
            n326 = event-data() -> ("VI Description"=w415:string)  [unwired: 1 in]
            n327 = Bundle(cluster=T26 {"VI Description"=""} ("Save VI Description Argument"), "VI Description"=w415) -> (w416:T26)
            n328 = call-poly <vilib>:"Delacor_lib_QMH_Enqueue Message (poly).vi"("Message Data"=w416, "Message"="Save VI Description", "Message Queue in"=w419) -> ("error out"=w422:errorcluster)  [unwired: 7 in, 1 out]
          }
          event User Event {
            # "Another Module called the \"Open Documentation\" API Method."
            n329 = event-data() -> ("Boolean"=w423:bool)  [unwired: 1 in]
            n330 = Bundle(cluster=T27 {"Boolean"=FALSE} ("Open Documentation Argument"), "Boolean"=w423) -> (w424:T27)
            n331 = call-poly <vilib>:"Delacor_lib_QMH_Enqueue Message (poly).vi"("Message Data"=w424, "Message"="Open Documentation", "Message Queue in"=w427) -> ("error out"=w430:errorcluster)  [unwired: 7 in, 1 out]
          }
          event "Open Antidoc Output": Value Change {
            # "Another Module called the \"Open Documentation\" API Method."
            n332 = event-data() -> ()  [unwired: 1 in, 1 out]
            n333 = Bundle(cluster=T27 {"Boolean"=FALSE} ("Open Documentation Argument"), "Boolean"="Open Antidoc Output") -> (w432:T27)
            n334 = call-poly <vilib>:"Delacor_lib_QMH_Enqueue Message (poly).vi"("Message Data"=w432, "Message"="Open Documentation", "Message Queue in"=w435) -> ("error out"=w438:errorcluster)  [unwired: 7 in, 1 out]
          }
          event User Event {
            # "Another Module called the \"Save Project Documentation\" API Method."
            n335 = event-data() -> ("Project Description"=w439:string)  [unwired: 1 in]
            n336 = Bundle(cluster=T28 {"Project Description"=""} ("Save Project Documentation Argument"), "Project Description"=w439) -> (w440:T28)
            n337 = call-poly <vilib>:"Delacor_lib_QMH_Enqueue Message (poly).vi"("Message Data"=w440, "Message"="Save Project Documentation", "Message Queue in"=w443) -> ("error out"=w446:errorcluster)  [unwired: 7 in, 1 out]
          }
          event User Event {
            # "Another Module called the \"Save Module Spec\" API Method."
            n338 = event-data() -> ("Boolean"=w448:bool)  [unwired: 1 in]
            n339 = Bundle(cluster=T29 {"Boolean"=FALSE} ("Save Module Spec Argument"), "Boolean"=w448) -> (w449:T29)
            n340 = call-poly <vilib>:"Delacor_lib_QMH_Enqueue Message (poly).vi"("Message Data"=w449, "Message"="Save Module Spec", "Message Queue in"=w452) -> ("error out"=w447:errorcluster)  [unwired: 7 in, 1 out]
          }
          event "Save Module Spec": Value Change {
            # "Another Module called the \"Save Module Spec\" API Method."
            n341 = event-data() -> ()  [unwired: 1 in, 1 out]
            n342 = Bundle(cluster=T29 {"Boolean"=FALSE} ("Save Module Spec Argument"), "Boolean"="Save Module Spec") -> (w457:T29)
            n343 = call-poly <vilib>:"Delacor_lib_QMH_Enqueue Message (poly).vi"("Message Data"=w457, "Message"="Save Module Spec", "Message Queue in"=w460) -> ("error out"=w456:errorcluster)  [unwired: 7 in, 1 out]
          }
        }
        n344 = call-dynamic "Delacor_lib_QMH_Error Handler - Event Handling Loop.vi"("error in"=w148, "Message Queue in"=w143) -> ("dup error in"=w147:errorcluster)  [unwired: 8 in, 1 out]
      }
      n345 = while {
        tunnel: w34 -> [w51]
        tunnel: [w50] -> w33
        shift-right: [w48] -> _
        shift-left: -1 -> [w47]
        shift-right: [w46] -> _
        shift-left: _ -> [w45]
        tunnel: w31 -> [w44]
        tunnel: [w52] -> w38
        shift-right: [w43] -> _
        shift-left: refnum<vi> refnum ("TreeControl out") -> [w42]
        stop <- w49 stop-if-true
        # "Helper Loop"
        n346 = event shown="[7] <Panther Dashboard Request Events.Register controls Mouse Enter>: User Event" {
          selector: w51 -> [_ _ _ _ _ _ _ w115 _ _ _]
          dyn-events: [_ _ _ _ _ _ _ w113 _ _ _] -> w50
          timeout: w47 -> [_ _ _ _ _ _ _ _ _ _ _]
          tunnel: [_ TRUE _ _ _ _ _ _ _ _ _] -> w49
          tunnel: [w55 w61 w67 w80 w92 w96 w108 w114 w122 w133 w137] -> w46
          tunnel: [w56 w62 500 w79 w91 w95 w107 w117 w121 w132 w136] -> w48
          tunnel: w47 -> [w56 w62 _ w79 w91 w95 w107 w117 w121 w132 w136]
          tunnel: w45 -> [w55 w61 _ w80 w92 w96 w108 w114 w122 w133 w137]
          tunnel: [w57 _ _ _ _ _ _ _ w123 _ _] -> w53
          tunnel: [w54 w59 w65 w78 w89 w94 w106 w116 w120 w131 w135] -> w43
          tunnel: w42 -> [w54 w59 _ w78 w89 w94 w106 w116 w120 w131 w135]
          event Timeout {
            n347 = event-data() -> ()  [unwired: 1 in, 1 out]
            n348 = call "Get Module Execution Status by ref.vi"("Modules Tree ref"=w54, "Refs"=w55) -> ("error out"=w57:errorcluster)  [unwired: 9 in]
          }
          event User Event {
            n349 = event-data() -> ()  [unwired: 1 in, 1 out]
            n350 = Unbundle By Name(w61) -> ("Modules"=w60:refnum<vi>[], "Application Instance"=w58:refnum<vi>)
            n351 = Close Reference(reference=w60) -> ()  [unwired: 1 in, 1 out]
            n352 = Close Reference(reference=w58) -> ()  [unwired: 1 in, 1 out]
          }
          event User Event {
            # "Refresh time"
            n353 = event-data() -> ("Modules"=w70:refnum<vi>[], "Modules Types"=w68:T9[], "Application Instance"=w69:refnum<vi>, "Dependencies"=w64:bool[])  [unwired: 1 in]
            n354 = Bundle By Name(cluster=T11 {"Modules"=[], "Modules Types"=[], "Application Instance"=refnum, "Dependencies"=[]}, "Modules"=w70, "Modules Types"=w68, "Application Instance"=w69, "Dependencies"=w64) -> (w67:T11)
            n355 = control-ref of="Modules Tree"() -> (w66:refnum<vi>)
            n356 = call "Set Tree custom symbols.vi"("TreeControl in"=w66) -> ("TreeControl out"=w65:refnum<vi>)  [unwired: 10 in]
          }
          event User Event {
            n357 = event-data() -> ("Projects"=w76:string[])  [unwired: 1 in]
            n358 = Array Size(array=w76) -> (size(s)=w75:i32)
            n359 = Equal?(x=1, y=w75) -> (x = y?=w73:bool)
            n360 = control-ref of="Projects"() -> (w77:refnum<vi>)
            n361 = case shown="False" w73 {
              tunnel: w77 -> [w83 w86]
              tunnel: w76 -> [w82 w85]
              frame True {
                n362 = Index Array(array=w82) -> (element=w81:string)  [unwired: 1 in]
                n363 = property class="CmbBox"(reference=w83, "Strings[]"=w82, "Val(Sgnl)"=w81) -> ()  [unwired: 1 in, 2 out]
              }
              frame False {
                n364 = property class="CmbBox"(reference=w86, "Strings[]"=w85, "Text.Text"="") -> ()  [unwired: 1 in, 2 out]
              }
            }
          }
          event User Event {
            n365 = event-data() -> ("Targets"=w88:string[])  [unwired: 1 in]
            n366 = Index Array(array=w88) -> (element=w87:string)  [unwired: 1 in]
            n367 = control-ref of="Targets"() -> (w90:refnum<vi>)
            n368 = property class="CmbBox"(reference=w90, "Strings[]"=w88, "Value"=w87) -> ()  [unwired: 1 in, 2 out]
          }
          event User Event {
            n369 = event-data() -> ("Progress"=→"Progress":u16)  [unwired: 1 in]
          }
          event Mouse Enter {
            n370 = event-data() -> ("CtlRef"=w97:refnum<vi>)  [unwired: 1 in]
            n371 = property class="Ctl"(reference=w97) -> ("Label.Text"=w103:string, "TipStrip"=w104:string)  [unwired: 1 in, 2 out]
            n372 = control-ref of="antidoc"() -> (w98:refnum<vi>)
            n373 = control-ref of="Panther Indicator"() -> (w102:refnum<vi>)
            n374 = control-ref of="Process Indicator"() -> (w101:refnum<vi>)
            n375 = control-ref of="Event Indicator"() -> (w100:refnum<vi>)
            n376 = Empty String/Path?(string/path=w104) -> (empty?=w105:bool)
            n377 = Build Array(w98, w102, w101, w100) -> (w99:refnum<vi>[])
            n378 = call "Set Indicators Visibility Status.vi"("Indicator Refs"=w99, "Label"=w103) -> ()  [unwired: 10 in]
            n379 = case shown="False" w105 {
              tunnel: w104 -> [w109 _]
              frame False {
                n380 = call "Status Updated.vi"("Status"=w109) -> ()  [unwired: 10 in, 1 out]
              }
              frame True {
              }
            }
          }
          event User Event {
            n381 = event-data() -> ()  [unwired: 1 in, 1 out]
            n382 = control-ref of="This VI"() -> (w111:refnum<vi>)
            n383 = property class="VI"(reference=w111) -> ("Panel"=w112:refnum<vi>)  [unwired: 1 in, 2 out]
            n384 = property class="Pnl"(reference=w112) -> ("Controls[]"=w110:refnum<vi>[])  [unwired: 1 in, 2 out]
            n385 = register-events(reference=w115, w110) -> (reference out=w113:refnum<event-registration>)  [unwired: 3 in, 1 out]
          }
          event User Event {
            n386 = event-data() -> ("Scale Max"=w119:i32)  [unwired: 1 in]
            n387 = control-ref of="Progress"() -> (w118:refnum<vi>)
            n388 = property class="Slide (strict)"(reference=w118, "Scale.Maximum"=w119) -> (error out=w123:errorcluster)  [unwired: 1 in, 1 out]
          }
          event User Event {
            n389 = event-data() -> ("Module Type"=w130:T9)  [unwired: 1 in]
            n390 = Equal?(x=Module_type--enum."Cloneable", y=w130) -> (x = y?=w128:bool)
            n391 = Select(t=T12."Enabled" ("Disabled"), s=w128, f=T12."Disabled and Grayed Out") -> (s? t:f=w125:T12)
            n392 = control-ref of="Module ID"() -> (w127:refnum<vi>)
            n393 = property class="DigNum (strict)"(reference=w127, "DisabledEnum"=w125) -> ()  [unwired: 1 in, 2 out]
          }
          event User Event {
            n394 = event-data() -> ("Status"=→"Status":string)  [unwired: 1 in]
          }
        }
        n395 = call-dynamic "Delacor_lib_QMH_Error Handler - Helper Loop.vi"("error in"=w53, "Message Queue in"=w44) -> ("dup error in"=w52:errorcluster)  [unwired: 8 in, 1 out]
      }
    }
    frame Error {
      # "Synchronize Caller Events.vi will inform Start Module.vi that the module has launched and will let the code calling Start Module.vi register for broadcasts and would permit the caller receive the broadcast that an error occurred at launch time."
      n396 = call-dynamic "Delacor_lib_QMH_Release Message Queue.vi"("error in"=w924, "Message Queue"=w918) -> ("error out"=w923:errorcluster)  [unwired: 9 in]
      n397 = call "Synchronize Caller Events.vi"("Singleton Module Admin in"=w919) -> ("error out"=w925:errorcluster)  [unwired: 9 in, 1 out]
      n398 = call "Module Name--constant.vi"() -> ("Module Name"=w921:string)  [unwired: 11 in]
      n399 = Format Into String(format string="An error occurred during initialization. %s is no longer running.", w921) -> (resulting string=w916:string)  [unwired: 2 in, 1 out]
      n400 = Merge Errors(w923, w925) -> (w926:errorcluster)
      n401 = call "Stop Module.vi"("Origin"=w916) -> ()  [unwired: 10 in, 1 out]
      n402 = call "Error Reported.vi"("Additional Information"=w916, "Error"=w926) -> ()  [unwired: 9 in, 1 out]
    }
  }
  n403 = Merge Errors(w24, w26, w19) -> (w23:errorcluster)
  n404 = call "Close Module.vi"("error in (no error)"=w23, "Module Admin in"=w14) -> ("error out"=w25:errorcluster, "External Launch"=w8:bool, "Module Admin out"=w9:refnum<class "Delacor_lib_QMH_Module Admin.lvclass">)  [unwired: 7 in]
  n405 = Unregister For Events(event registration refnum=w6) -> ()  [unwired: 1 in, 1 out]
  n406 = Unregister For Events(event registration refnum=w13, error in=w25) -> (error out=w22:errorcluster)
  "error out" <- w22
  n407 = case "External Launch?" shown="True" w8 {
    tunnel: w22 -> [_ w927]
    frame False {
    }
    frame True {
      n408 = case shown="No Error" w927 {
        frame No Error {
          n409 = invoke class="VI" method="FP.Close"() -> ()  [unwired: 3 in, 3 out]
        }
        frame Error {
          n410 = invoke on="Invoke Node" class="VI" method="FP.Open"("Activate"=TRUE ("Activate?")) -> ()  [unwired: 4 in, 5 out]
        }
      }
    }
  }
  n411 = local write "Module Admin"(w9) -> ()
